vi "Set_Control_Parameter.vi"(0 "Set Mode":T18, 1 "Settings ok? in":bool, 5 "Settings message":T16, 7 "Main Parameters in":T1={"Mode"={"Mode"=enum."Dialog", "Expert?"=FALSE, "Dialog?"=FALSE}, "Stop loop"={"Settings changed?"=FALSE, "Stop?"=refnum}, "Send message"={"Send mode"=enum."Get parameters", "Set parameter list"=0, "Get parameter list"=0, "Reset device"=0, "Length set settings message"=0, "Reset buttons?"=FALSE, "Reset Master?"=enum."General"}, "Write settings"={"Options"=enum."File 1"}, "Settings state"={"MAS locked?"=refnum, "SLV locked?"=refnum}, "Button refs"={"Stop program"=refnum, "Save settings"=refnum, "DAQ mode"=refnum, "Reset settings"=refnum, "Apply settings"=refnum, "Reset MAS"=refnum, "Reset SLV"=refnum, "Local DBase?"=refnum, "Last value DBase"=FALSE, "Database"=refnum, "Calibration"=refnum, "Save settings 2"=refnum}, "Update screen"={"Detector number"=0, "Hardware"=enum."None"}, "Files"={"Path config file"=path "", "Path def. ini file"=path "", "Path ini file 1"=path "", "Path ini file 2"=path "", "Path RBF file"=path ""}, "DB connection"={"connection reference"=refnum, "Connected?"=refnum, "ODBC Name"=""}, "Status_id"=refnum, "Time difference"=refnum, "Satellites"=refnum, "Alignment parameters"=refnum, "Page Statistics 2"=refnum, "Database"=refnum, "Page Statistics"=refnum} {"Update screen"."Detector number" format="%#.0f"; "Send message"."Reset device" format="%x"; "Send message"."Get parameter list" format="%x"; "Send message"."Set parameter list" format="%x"}, 9 "Control Parameter in":T15 {"Aux Byte Value" format="%02x"; "Max Real Value" format="%#_6e"; "Min Real Value" format="%#_6e"; "dReal/dByte" format="%#_6e"; "Byte Value" format="%02x"; "Identifier" format="%02x"}, 11 "Status/Errors in":refnum<vi>, 12 "Control Parameters [] in":T15[](array[typedef]) {"Aux Byte Value" format="%02x"; "Max Real Value" format="%#_6e"; "Min Real Value" format="%#_6e"; "dReal/dByte" format="%#_6e"; "Byte Value" format="%02x"; "Identifier" format="%02x"}, 14 "Set value from device (f)":bool) -> (3 "Settings ok? out":bool, 4 "Value Changed?":bool, 8 "Run twice?":bool, 10 "Control Parameter out":T15 {"Aux Byte Value" format="%02x"; "Max Real Value" format="%#_6e"; "Min Real Value" format="%#_6e"; "dReal/dByte" format="%#_6e"; "Byte Value" format="%02x"; "Identifier" format="%02x"}, 15 "Status/Errors out":refnum<vi>)   [LabVIEW 2010]
uses:
  Controls/Control_Parameters.ctl
  Controls/Master.ctl
  Controls/Set_Mode.ctl
  Controls/Settings_Message.ctl
  Controls/Setting.ctl
  Controls/Main_Parameters.ctl
  Controls/Mode.ctl
  Controls/Stop_Loop.ctl
  Controls/Send_Message.ctl
  Controls/Send_Message_Mode.ctl
  Controls/Write_Settings.ctl
  Controls/Write_Settings_Options.ctl
  Controls/Settings_State.ctl
  Controls/Button_Refs.ctl
  Controls/Update_Screen.ctl
  Controls/Files.ctl
  Controls/DB_Connection.ctl
  database/Connection.llb/Conn ObjectReference.ctl
  Controls/TabPage_TriggerConditon.ctl
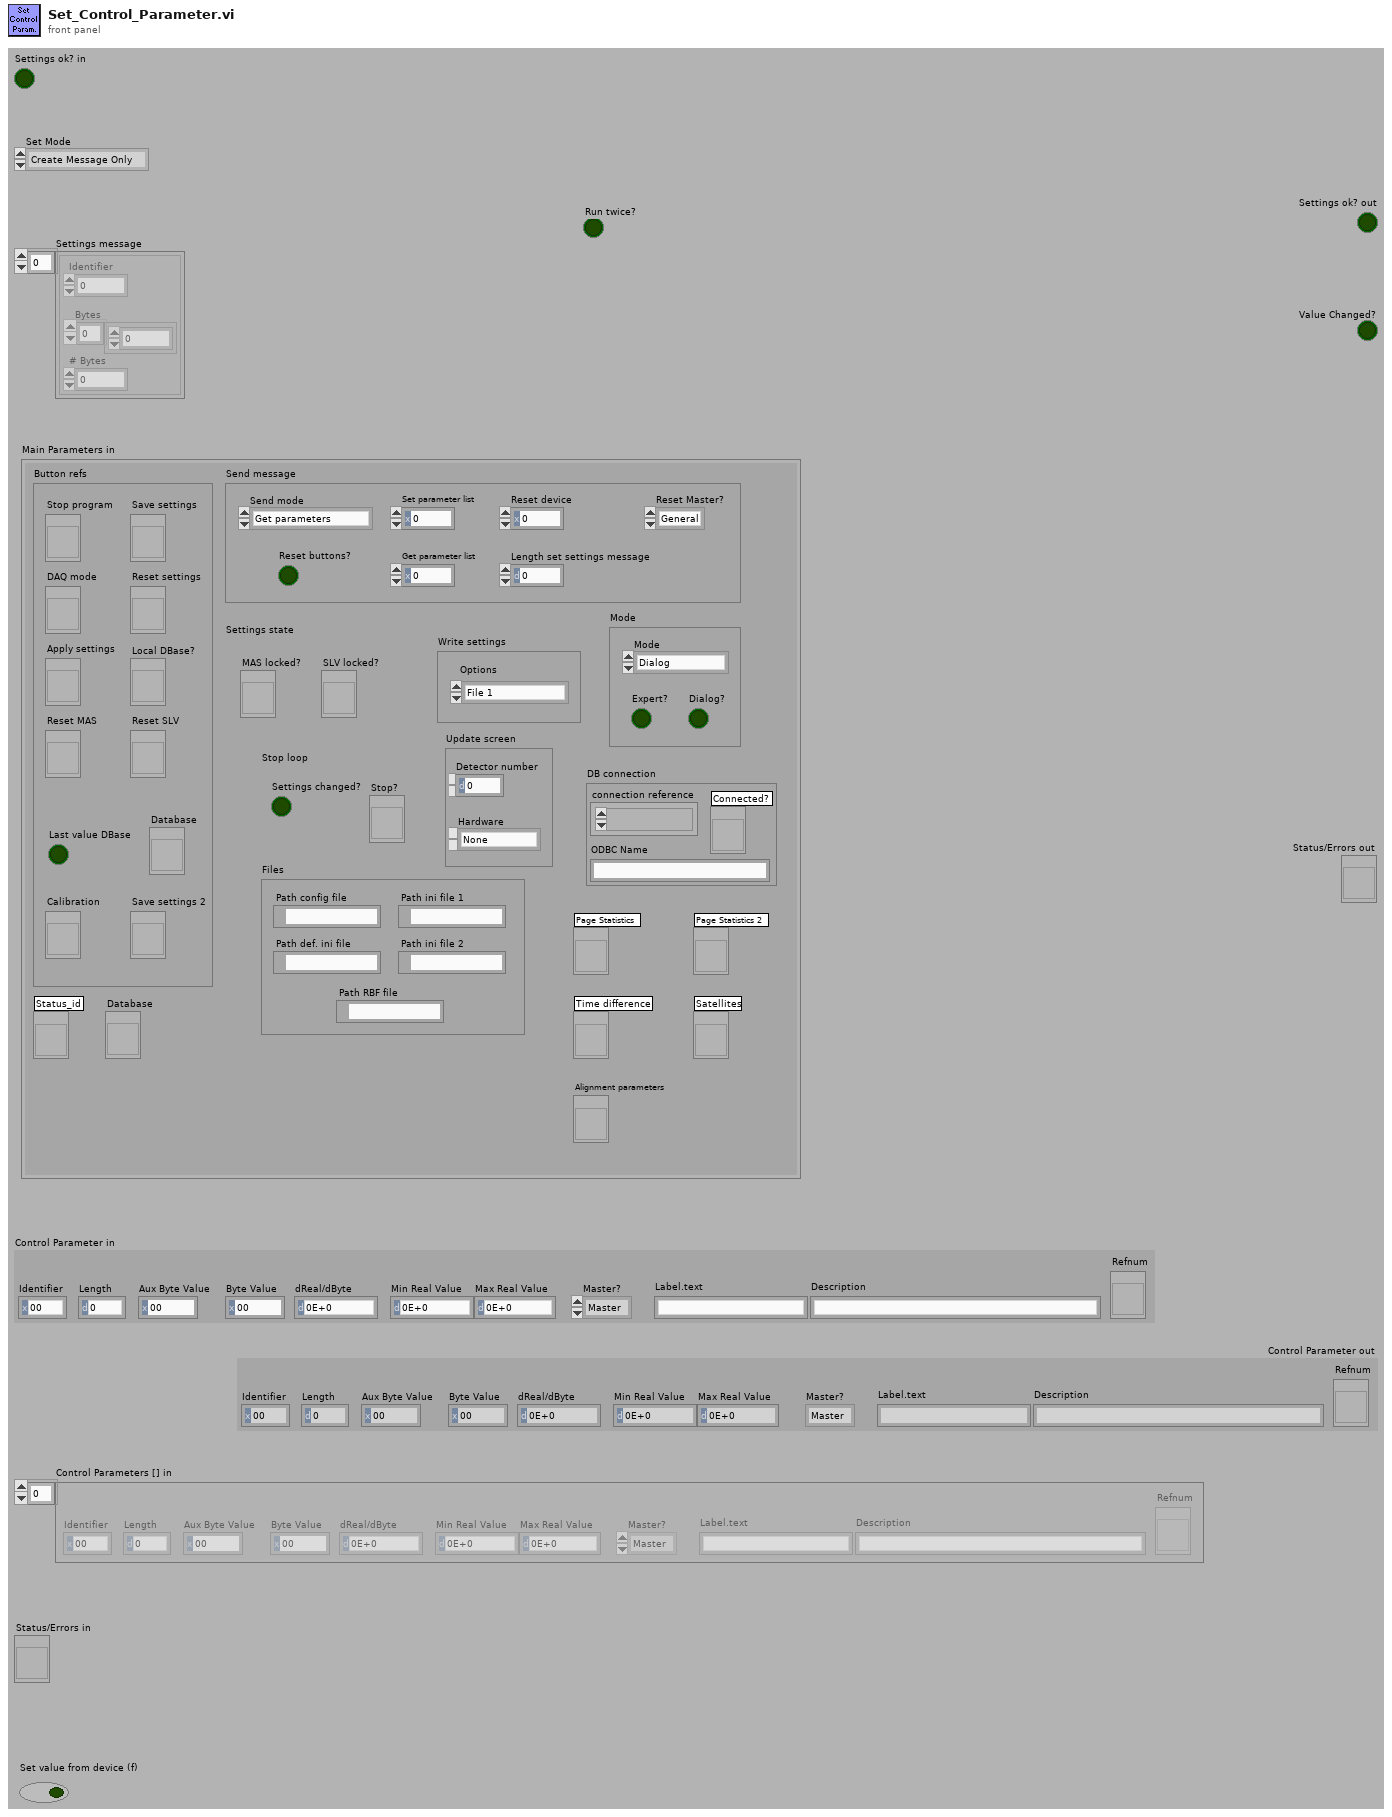
[diagram p1: front panel]
types:
  T1 = typedef "Main_Parameters.ctl" = cluster{"Mode":T2, "Stop loop":T3, "Send message":T4, "Write settings":T7, "Settings state":T9, "Button refs":T10, "Update screen":T11, "Files":T12, "DB connection":T13, "Status_id":refnum<vi>, "Time difference":refnum<vi>, "Satellites":refnum<vi>, "Alignment parameters":refnum<vi>, "Page Statistics 2":refnum<vi>, "Database":refnum<vi>, "Page Statistics":refnum<vi>}
  T2 = typedef "Mode.ctl" = cluster{"Mode":enum8{"Stop", "Dialog", "Hisparc II", "Hisparc II DAQ", "Alignment"}, "Expert?":bool, "Dialog?":bool}
  T3 = typedef "Stop_Loop.ctl" = cluster{"Settings changed?":bool, "Stop?":refnum<vi>}
  T4 = typedef "Send_Message.ctl" = cluster{"Send mode":T5, "Set parameter list":u8, "Get parameter list":u8, "Reset device":u8, "Length set settings message":i32, "Reset buttons?":bool, "Reset Master?":T6}
  T5 = typedef "Send_Message_Mode.ctl" = enum16{"Get parameters", "Set parameters", "From front panel", "From parameters", "Reset device", "Alignment"}
  T6 = typedef "Master.ctl" = enum16{"Master", "Slave", "General"}
  T7 = typedef "Write_Settings.ctl" = cluster{"Options":T8}
  T8 = typedef "Write_Settings_Options.ctl" = enum16{"File 1", "File 2", "Alignment", "Reset"}
  T9 = typedef "Settings_State.ctl" = cluster{"MAS locked?":refnum<vi>, "SLV locked?":refnum<vi>}
  T10 = typedef "Button_Refs.ctl" = cluster{"Stop program":refnum<vi>, "Save settings":refnum<vi>, "DAQ mode":refnum<vi>, "Reset settings":refnum<vi>, "Apply settings":refnum<vi>, "Reset MAS":refnum<vi>, "Reset SLV":refnum<vi>, "Local DBase?":refnum<vi>, "Last value DBase":bool, "Database":refnum<vi>, "Calibration":refnum<vi>, "Save settings 2":refnum<vi>}
  T11 = typedef "Update_Screen.ctl" = cluster{"Detector number":u16, "Hardware":enum8{"None", "HiSPARC I", "HiSPARC II", "HiSPARC III", "Unknown"}}
  T12 = typedef "Files.ctl" = cluster{"Path config file":path, "Path def. ini file":path, "Path ini file 1":path, "Path ini file 2":path, "Path RBF file":path}
  T13 = typedef "DB_Connection.ctl" = cluster{"connection reference":T14, "Connected?":refnum<vi>, "ODBC Name":string}
  T14 = typedef "Conn ObjectReference.ctl" = refnum<k1>
  T15 = typedef "Control_Parameters.ctl" = cluster{"Identifier":u8, "Length":u16, "Byte Value":u32, "dReal/dByte":dbl, "Min Real Value":dbl, "Max Real Value":dbl, "Master?":T6, "Label.text":string, "Description":string, "Refnum":refnum<vi>, "Aux Byte Value":u32}
  T16 = typedef "Settings_Message.ctl" = T17[]
  T17 = typedef "Setting.ctl" = cluster{"Identifier":u8, "  Bytes":u8[], "# Bytes":u16}
  T18 = typedef "Set_Mode.ctl" = enum16{"Create Message Only", "Front Panel", "Parameters", "Master", "Slave"}
  T19 = cluster{"Filter_Data":bool, "Use_Thresh":bool, "Reduce data?":bool}
  T20 = typedef "TabPage_TriggerConditon.ctl" = cluster{"# low signals":enum32{"no low", "1 low", "2 low", "3 low", "4 low"}, "# high signals":enum32{"no high", "1 high", "2 high", "3 high", "4 high"}, "External trigger":enum32{"no ext", "with ext", "only ext"}, "And_Or":cluster{"Switch":bool}}
  T21 = enum32{"no low", "1 low", "2 low", "3 low", "4 low"}
  T22 = enum32{"no high", "1 high", "2 high", "3 high", "4 high"}
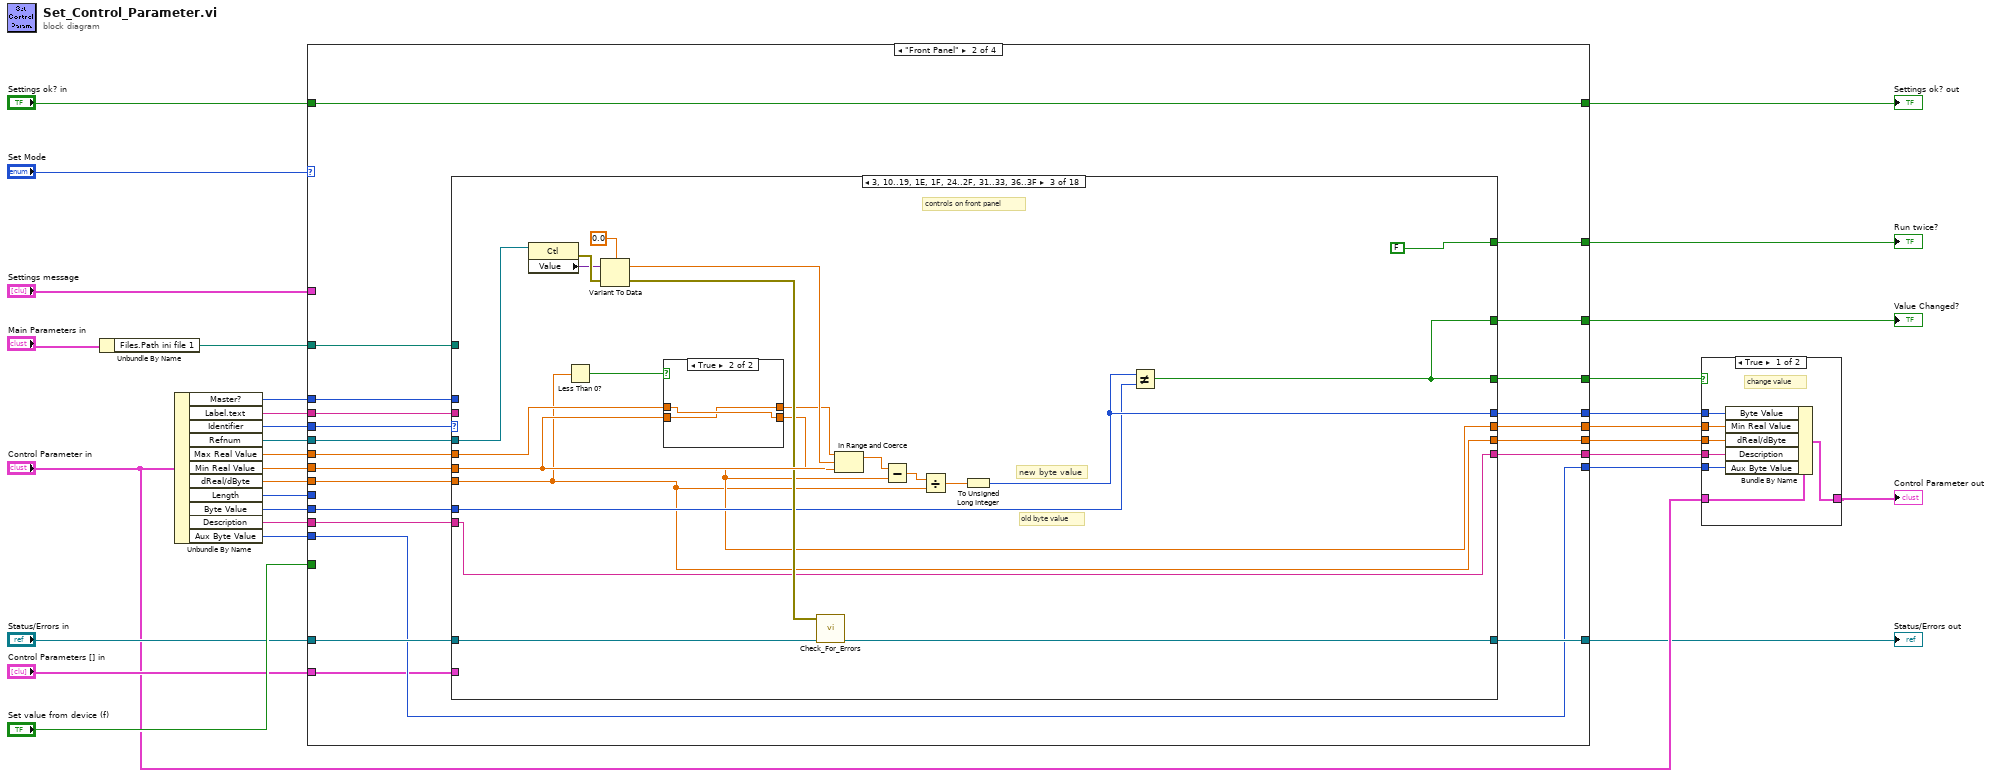
[diagram p0: block diagram]
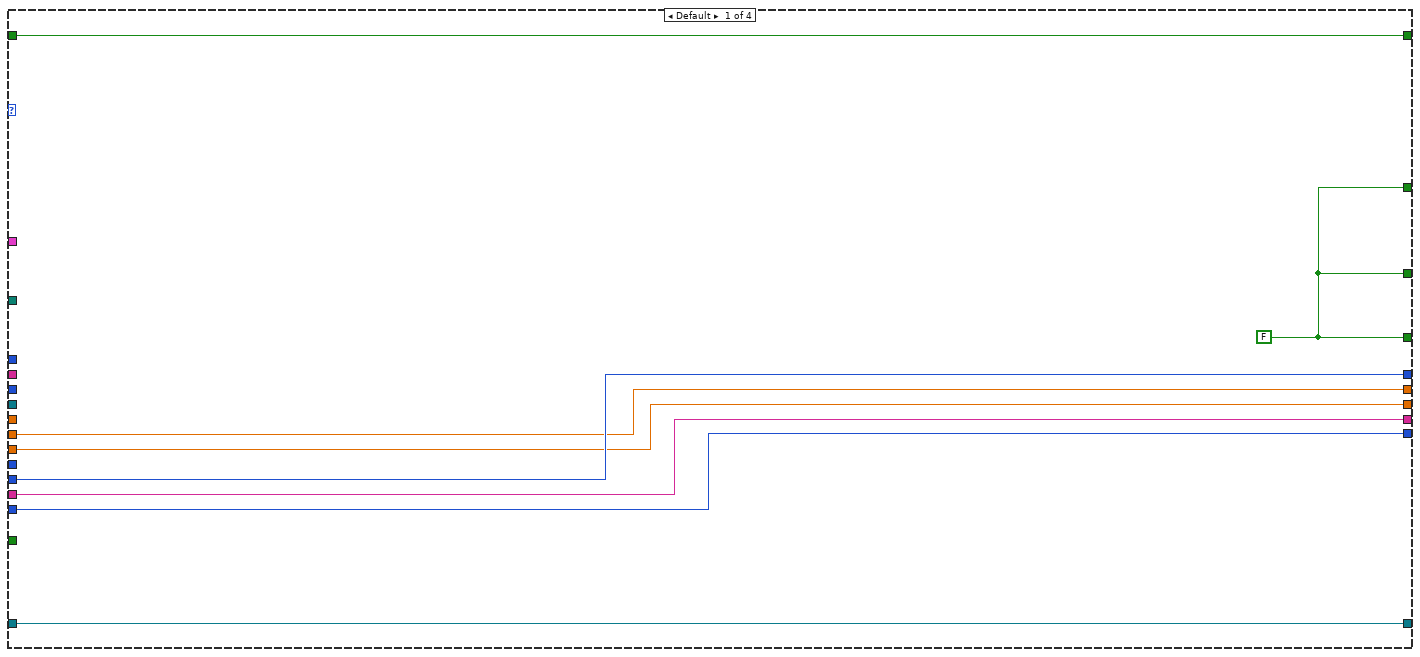
[diagram p3: hidden frame]
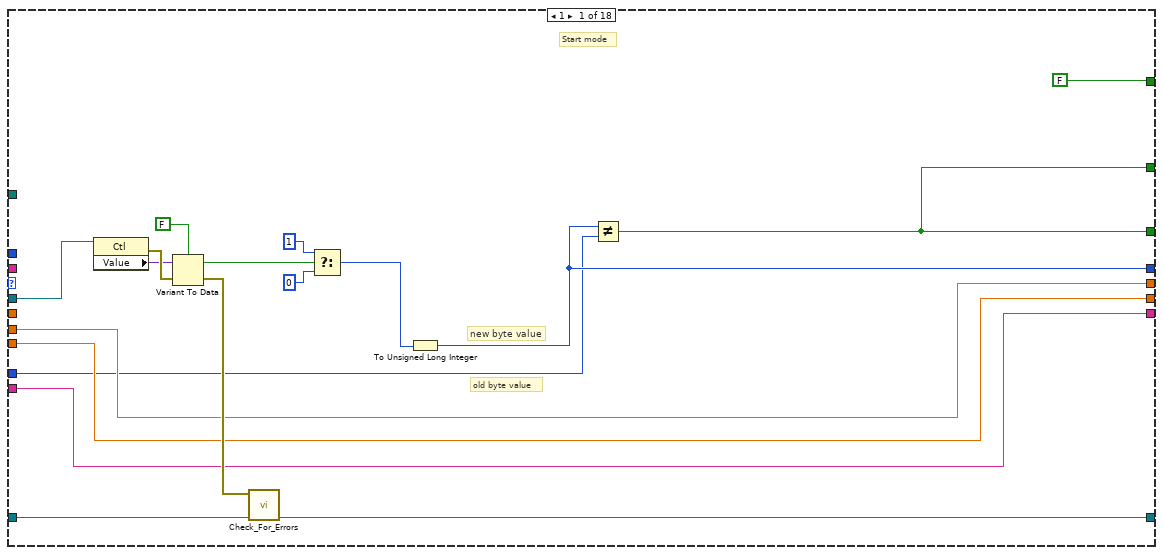
[diagram p4: hidden frame]
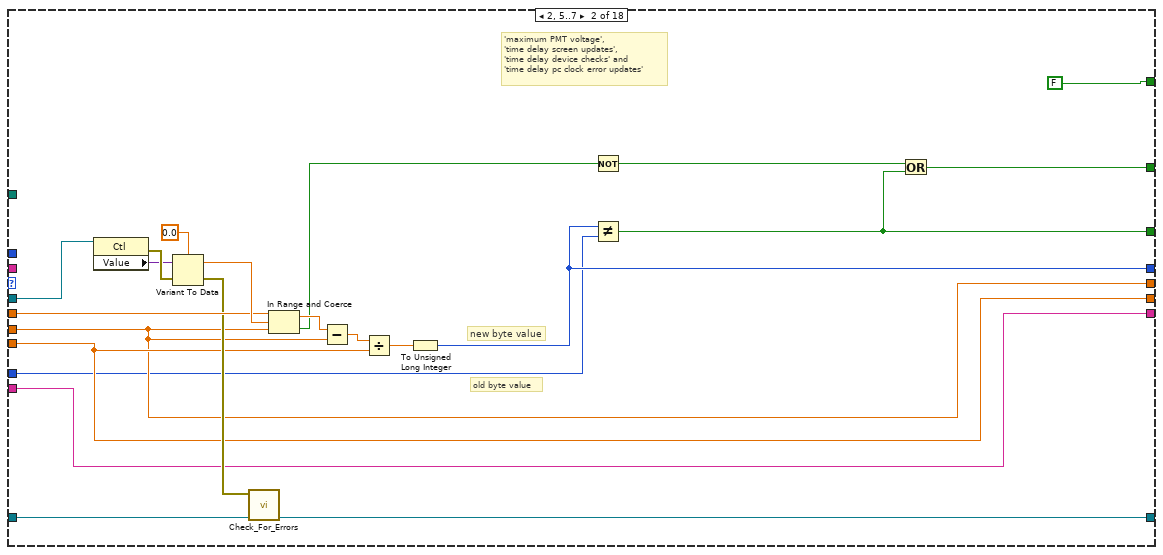
[diagram p5: hidden frame]
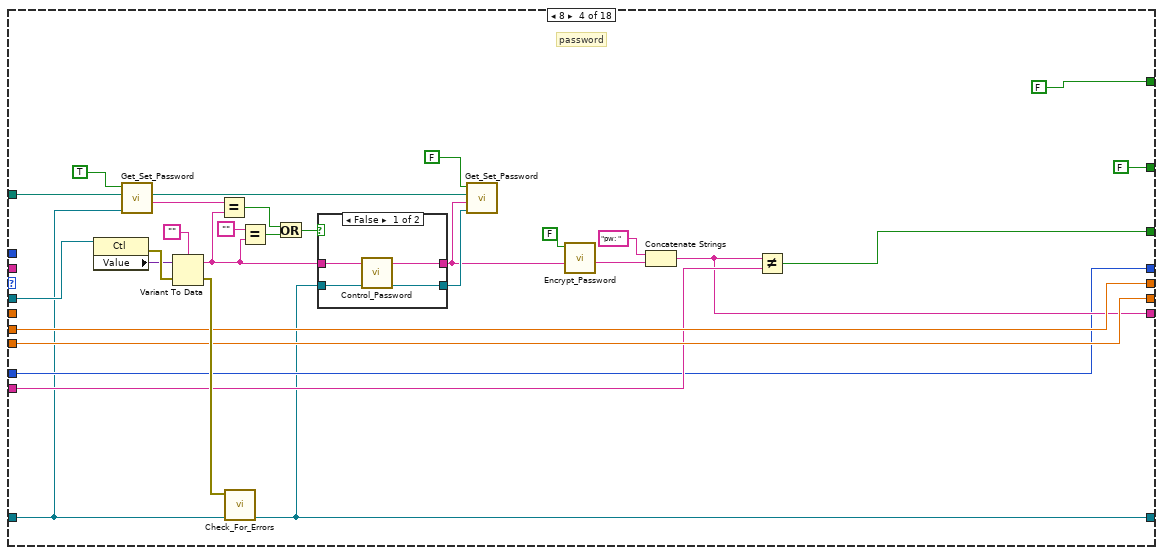
[diagram p7: hidden frame]
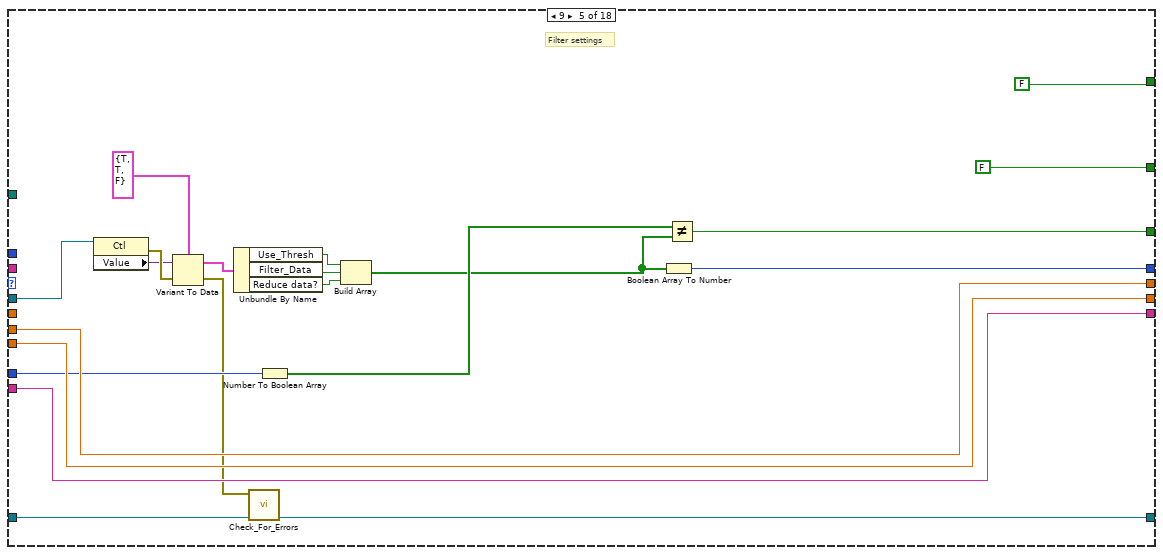
[diagram p9: hidden frame]
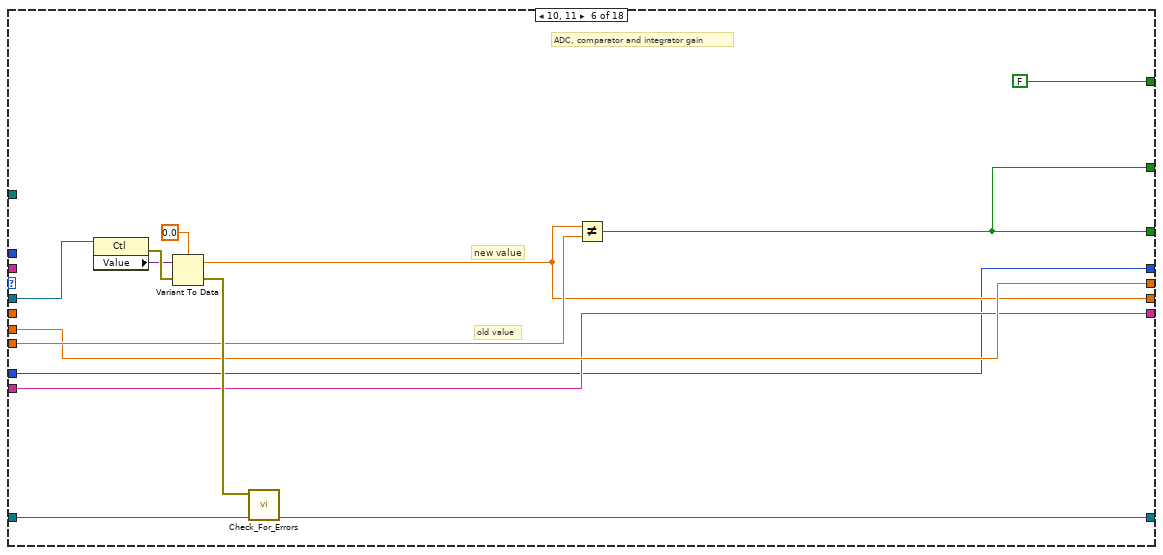
[diagram p10: hidden frame]
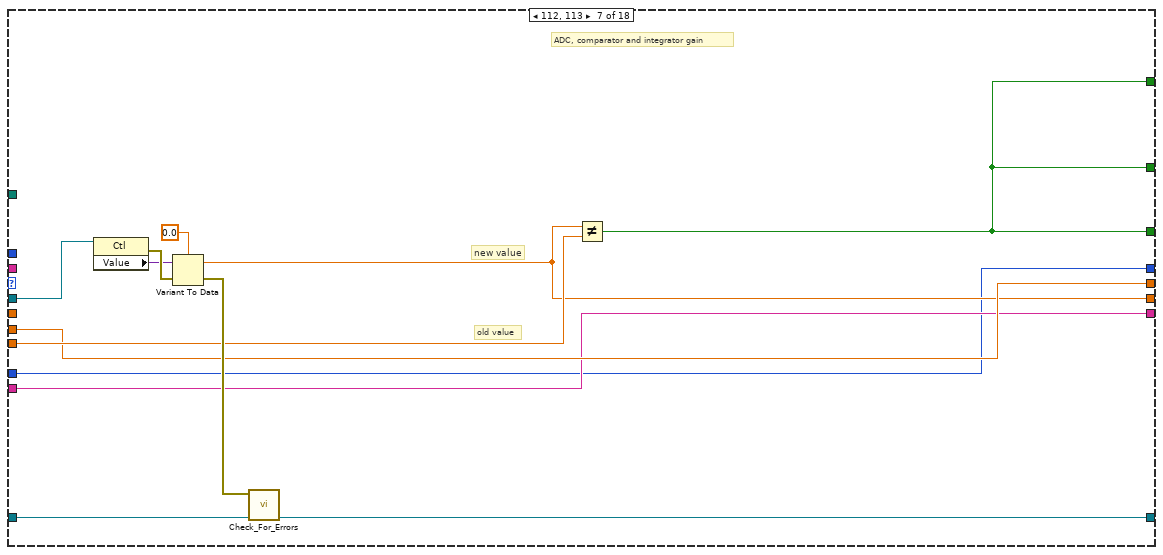
[diagram p11: hidden frame]
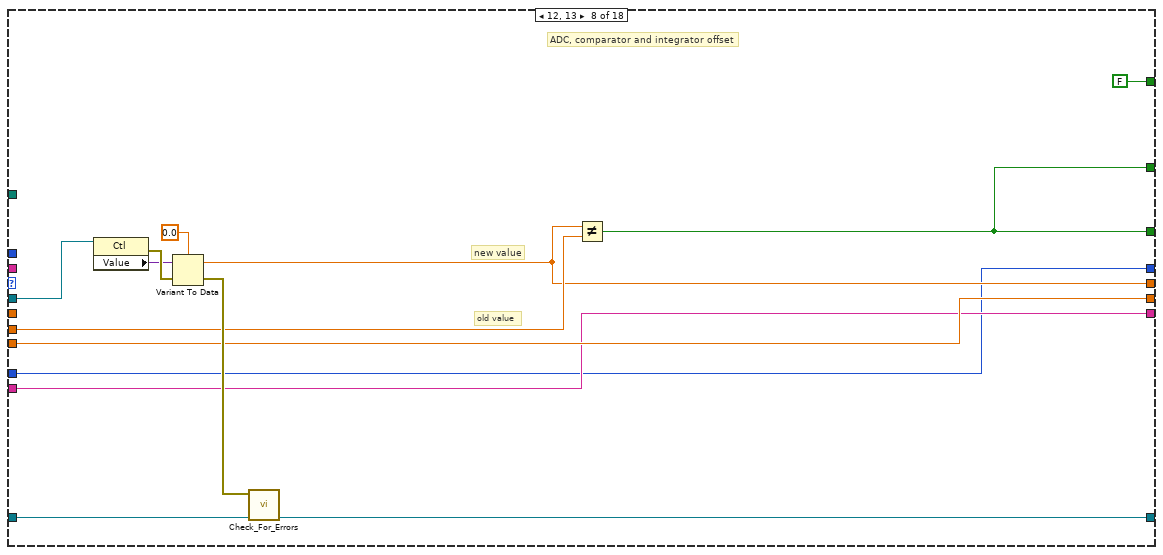
[diagram p12: hidden frame]
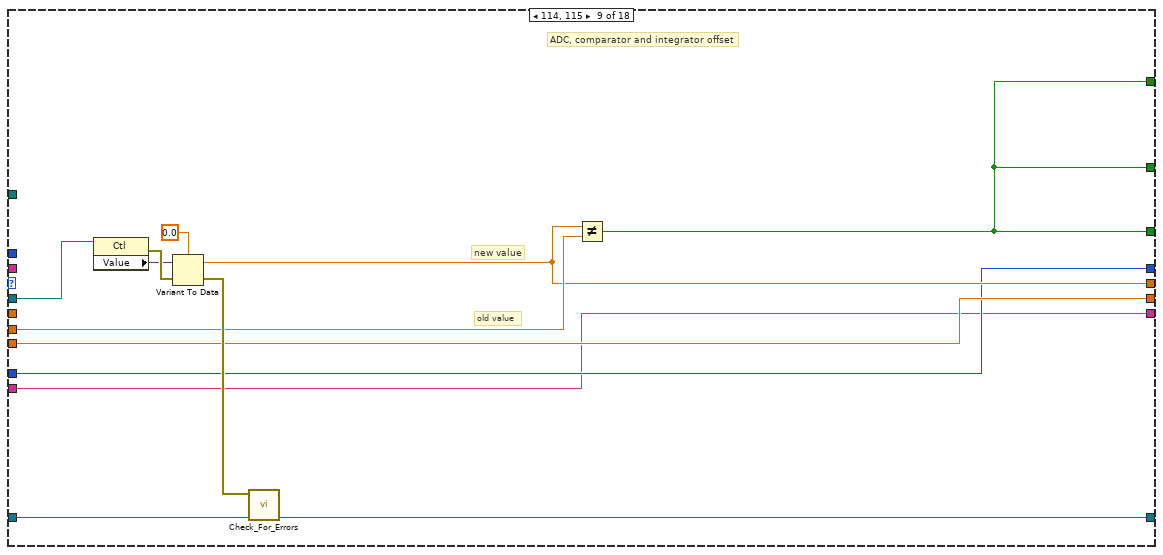
[diagram p13: hidden frame]
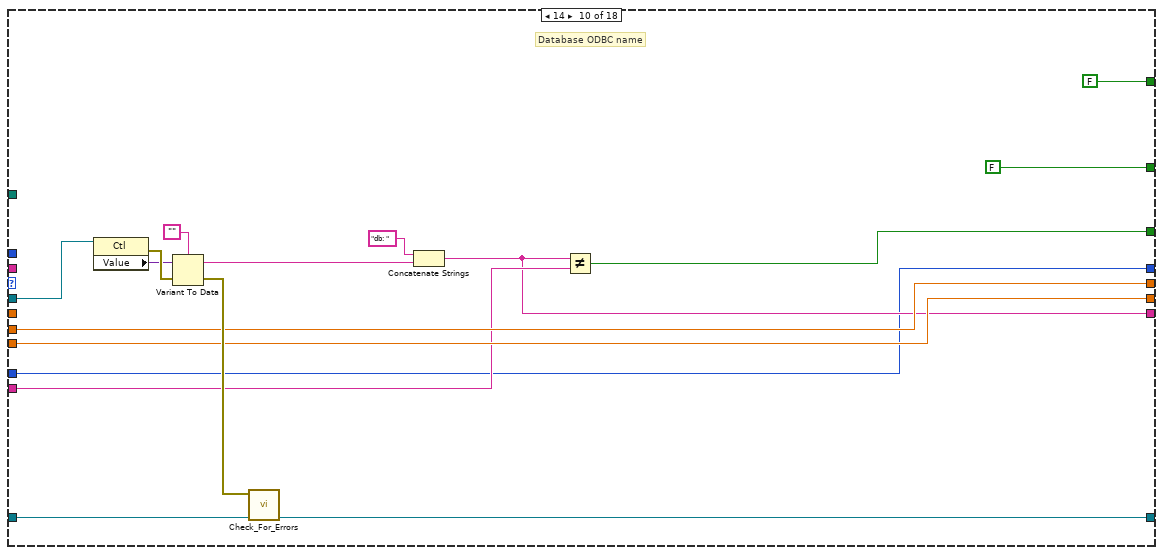
[diagram p14: hidden frame]
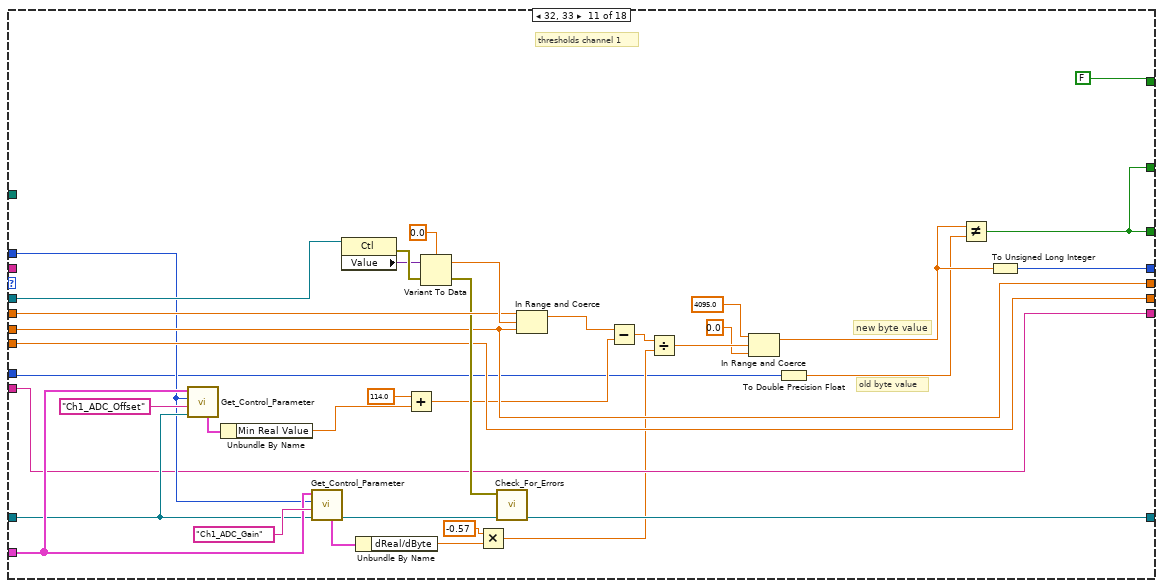
[diagram p15: hidden frame]
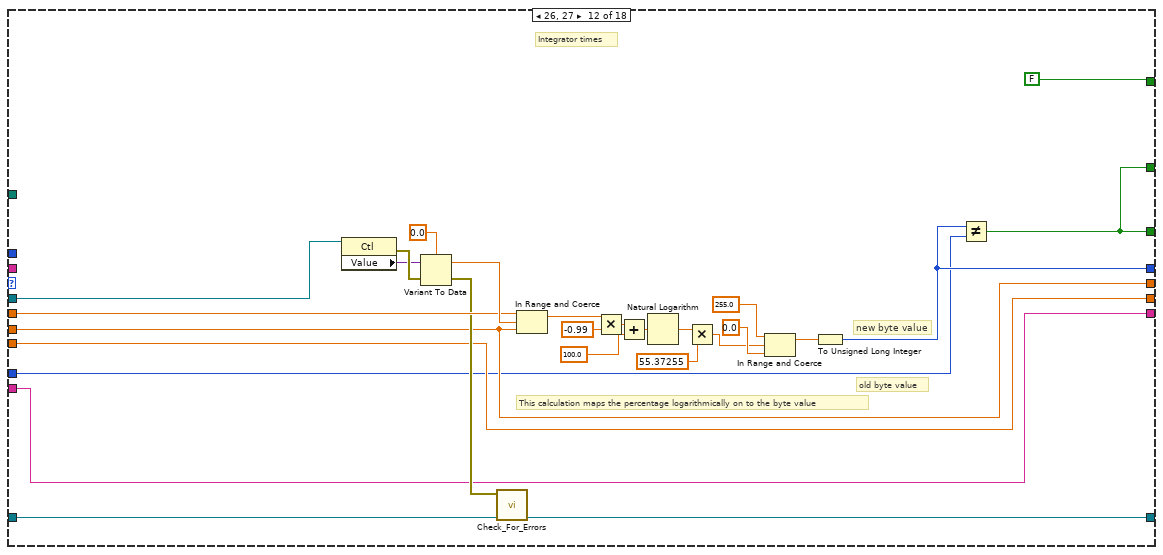
[diagram p16: hidden frame]
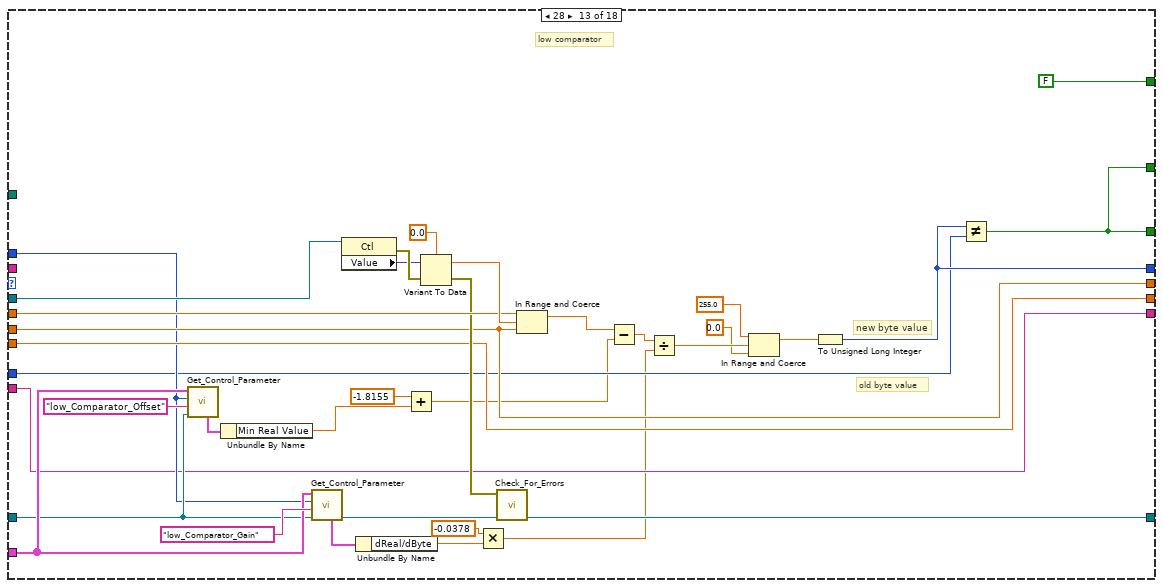
[diagram p17: hidden frame]
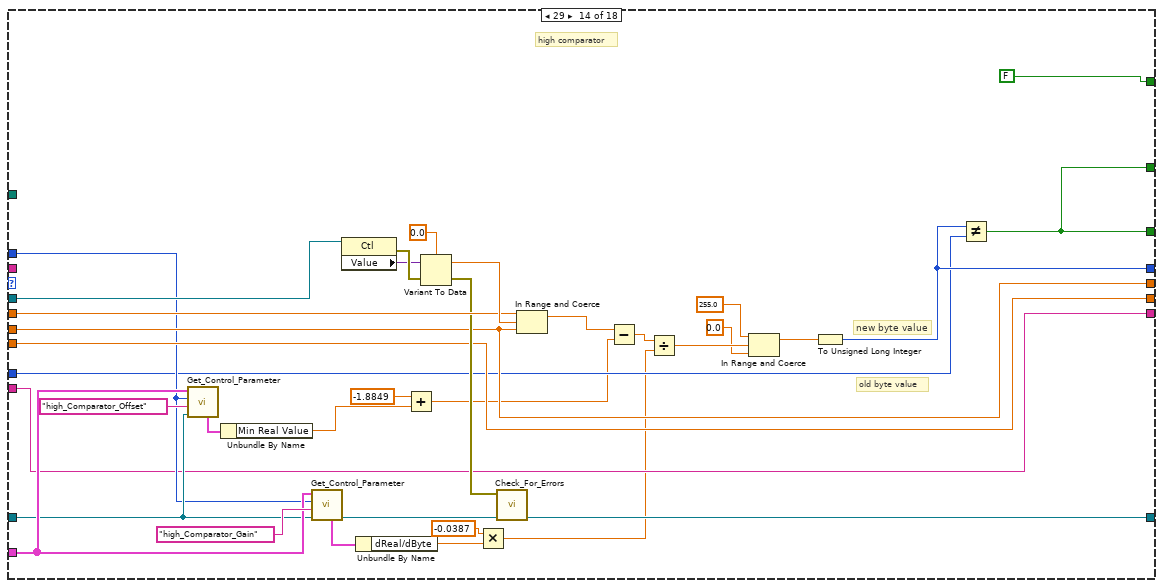
[diagram p18: hidden frame]
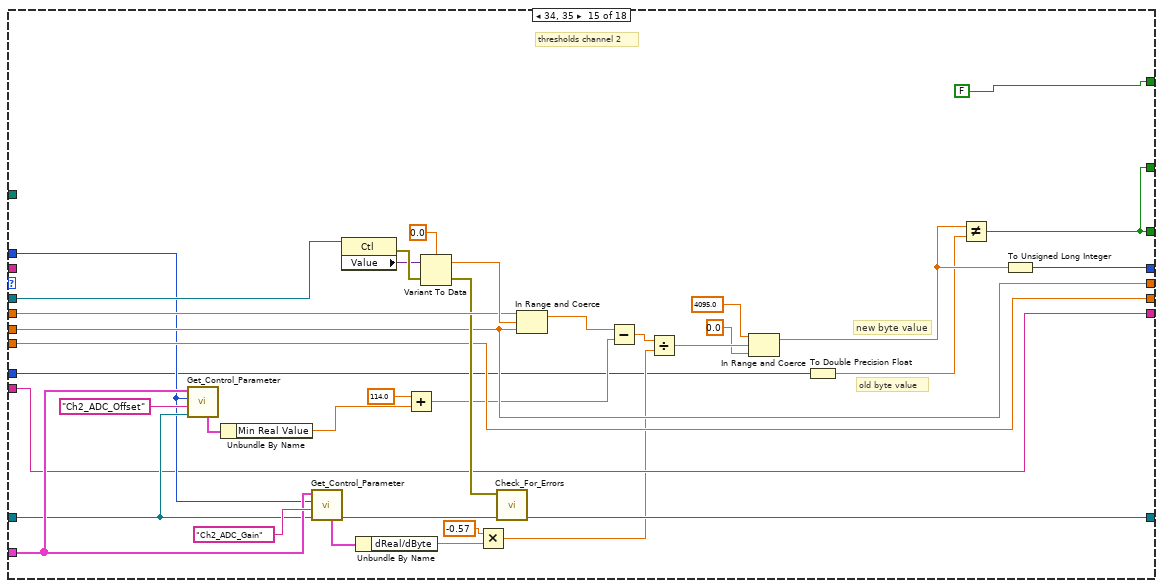
[diagram p19: hidden frame]
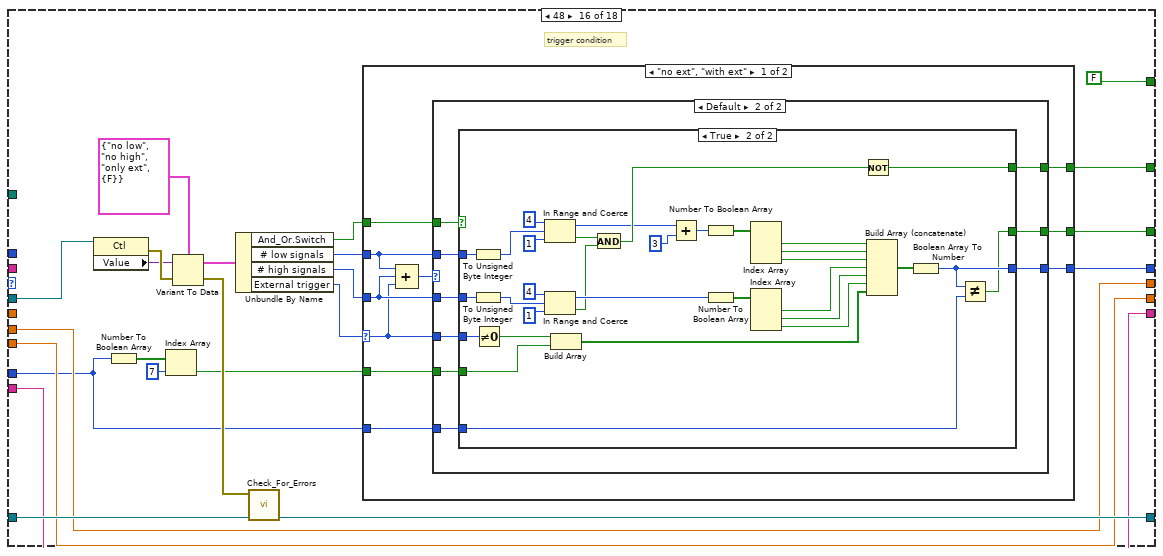
[diagram p20: hidden frame]
diagram:
  n1 = Unbundle By Name("Main Parameters in") -> ("Files.Path ini file 1"=w5:path)
  n2 = Unbundle By Name("Control Parameter in") -> ("Master?"=w24:T6, "Label.text"=w23:string, "Identifier"=w22:u8, "Refnum"=w21:refnum<vi>, "Max Real Value"=w20:dbl, "Min Real Value"=w19:dbl, "dReal/dByte"=w18:dbl, "Length"=w17:u16, "Byte Value"=w16:u32, "Description"=w15:string, "Aux Byte Value"=w14:u32)
  n3 = case shown="\"Front Panel\"" "Set Mode" {
    selector: "Set Mode" -> [_ _ w582 w855]
    tunnel: w19 -> [w34 w61 w567 w839]
    tunnel: w18 -> [w35 w60 w568 w840]
    tunnel: w16 -> [w39 w43 w585 w858]
    tunnel: [w38 w56 w578 w851] -> w1
    tunnel: w21 -> [_ w59 _ _]
    tunnel: w22 -> [_ w57 w574 w847]
    tunnel: w20 -> [_ w58 _ _]
    tunnel: "Settings message" -> [_ _ w584 w857]
    tunnel: w23 -> [_ w49 w581 w854]
    tunnel: w24 -> [_ w50 w580 w853]
    tunnel: [w39 w54 w579 w852] -> w30
    tunnel: [w32 w55 w570 w843] -> w28
    tunnel: "Status/Errors in" -> [w38 w53 w578 w851]
    tunnel: w17 -> [_ _ w577 w850]
    tunnel: [w37 w41 w576 w849] -> w3
    tunnel: "Settings ok? in" -> [w37 w41 w575 w848]
    tunnel: w14 -> [w36 w52 w572 w845]
    tunnel: [w36 w52 w571 w844] -> w29
    tunnel: [w32 w51 w570 w843] -> w4
    tunnel: "Set value from device (f)" -> [_ _ w569 w842]
    tunnel: [w34 w48 w567 w839] -> w27
    tunnel: [w35 w47 w568 w840] -> w25
    tunnel: "Control Parameters [] in" -> [_ w46 _ _]
    tunnel: w15 -> [w33 w45 w566 w841]
    tunnel: [w33 w44 w566 w841] -> w26
    tunnel: w5 -> [_ w42 _ _]
    tunnel: [w32 w40 FALSE FALSE] -> w2
    frame Default {
      w32 = FALSE
    }
    frame "Front Panel" {
      n4 = case shown="3, 10..19, 1E, 1F, 24..2F, 31..33, 36..3F" w57 {
        tunnel: w61 -> [w71 w83 w107 w151 w182 w190 w203 w218 w231 w247 w282 w309 w343 w378 w415 w429 w553 w563]
        tunnel: w60 -> [w70 w84 w105 w152 w183 w191 w204 w217 w230 w248 w281 w308 w342 w377 w414 w430 w554 w562]
        tunnel: w53 -> [w74 w91 w114 w140 w176 w193 w206 w220 w233 w250 w275 w302 w336 w371 w408 w443 w545 w564]
        tunnel: [w73 w85 w113 w141 w175 w192 w205 w219 w232 w249 w283 w311 w345 w380 w416 w442 w545 w564] -> w56
        tunnel: w59 -> [w76 w94 w116 w154 w174 w195 w208 w222 w235 w252 w286 w314 w348 w383 w419 w445 _ _]
        tunnel: w58 -> [_ w93 w106 _ _ _ _ _ _ _ w285 w313 w347 w382 w418 _ _ _]
        tunnel: [w65 w87 w102 w145 w167 w186 w199 w213 w226 w243 w260 w292 w319 w354 w393 w434 w558 w559] -> w55
        tunnel: [w72 w88 w112 w143 w168 w187 w200 w214 w228 w241 w259 w310 w344 w379 w392 w433 w556 w560] -> w54
        tunnel: [w65 w86 w102 FALSE FALSE w186 w199 w213 w226 FALSE w260 w292 w319 w354 w393 w435 FALSE w559] -> w51
        tunnel: w50 -> [_ _ _ _ _ _ _ _ _ _ w273 _ w334 w369 w406 _ _ _]
        tunnel: w49 -> [_ _ _ _ _ _ _ _ _ _ _ _ _ _ _ _ _ _]
        tunnel: [w71 w83 w107 w151 w182 w190 w203 w216 w229 w247 w282 w309 w343 w378 w415 w429 w553 w563] -> w48
        tunnel: [w70 w84 w105 w152 w183 w189 w202 w217 w230 w248 w281 w308 w342 w377 w414 w430 w554 w562] -> w47
        tunnel: w46 -> [_ _ _ _ _ _ _ _ _ _ w276 _ w337 w372 w409 _ _ _]
        tunnel: w45 -> [w64 w82 w111 w147 w181 w188 w201 w215 w227 w245 w272 w307 w333 w368 w405 w428 w548 w561]
        tunnel: [w64 w82 w111 w146 w181 w188 w201 w215 w227 w244 w272 w307 w333 w368 w405 w428 w548 w561] -> w44
        tunnel: w43 -> [w63 w81 w110 w143 w180 w187 w200 w214 w228 w241 w256 w306 w332 w367 w390 w427 w547 w560]
        tunnel: w42 -> [_ _ _ w138 _ _ _ _ _ _ _ _ _ _ _ _ _ _]
        tunnel: [FALSE FALSE FALSE FALSE FALSE FALSE w199 FALSE w226 FALSE FALSE FALSE FALSE FALSE FALSE FALSE FALSE w559] -> w40
        frame 1 {
          # "Start mode"
          # "old byte value"
          # "new byte value"
          n5 = property class="Ctl"(reference=w76) -> (error out=w79:errorcluster, "Value"=w78:variant)  [unwired: 1 in, 1 out]
          n6 = Variant To Data(error in=w79, Variant=w78, type=FALSE) -> (error out=w75:errorcluster, data=w69:bool)
          n7 = call "Check_For_Errors.vi"("Status/Errors in"=w74, "error in"=w75) -> ("Status/Errors out"=w73:refnum<vi>)  [unwired: 9 out]
          n8 = Select(t=u32 1 ("number"), s=w69, f=u32 0 ("number")) -> (s? t:f=w66:u32)
          n9 = To Unsigned Long Integer(number=w66) -> (unsigned 32bit integer=w72:u32)
          n10 = Not Equal?(x=w72, y=w63) -> (x != y?=w65:bool)
        }
        frame 2, 5..7 {
          # "old byte value"
          # "new byte value"
          # "'maximum PMT voltage',\n'time delay screen updates',\n'time delay device checks' and\n'time delay pc clock error updates'"
          n11 = property class="Ctl"(reference=w94) -> (error out=w101:errorcluster, "Value"=w100:variant)  [unwired: 1 in, 1 out]
          n12 = Variant To Data(error in=w101, Variant=w100, type=0.0 ("Byte Value")) -> (error out=w92:errorcluster, data=w98:dbl)
          n13 = call "Check_For_Errors.vi"("Status/Errors in"=w91, "error in"=w92) -> ("Status/Errors out"=w85:refnum<vi>)  [unwired: 9 out]
          n14 = In Range and Coerce(upper limit=w93, x=w98, lower limit=w83) -> (coerced(x)=w97:dbl, In Range?=w89:bool)
          n15 = Subtract(x=w97, y=w83) -> (x-y=w96:dbl)
          n16 = Divide(x=w96, y=w84) -> (x/y=w95:dbl)
          n17 = To Unsigned Long Integer(number=w95) -> (unsigned 32bit integer=w88:u32)
          n18 = Not(x=w89) -> (.not. x?=w90:bool)
          n19 = Not Equal?(x=w88, y=w81) -> (x != y?=w87:bool)
          n20 = Or(x=w90, y=w87) -> (x .or. y?=w86:bool)
        }
        frame 3, 16..25, 30, 31, 36..47, 49..51, 54..63 {
          # "old byte value"
          # "new byte value"
          # "controls on front panel"
          n21 = property class="Ctl"(reference=w116) -> (error out=w123:errorcluster, "Value"=w122:variant)  [unwired: 1 in, 1 out]
          n22 = Less Than 0?(x=w105) -> (x < 0?=w104:bool)
          n23 = Variant To Data(error in=w123, Variant=w122, type=0.0 ("Byte Value")) -> (error out=w115:errorcluster, data=w120:dbl)
          n24 = case shown="True" w104 {
            tunnel: w106 -> [w125 w127]
            tunnel: w107 -> [w124 w126]
            tunnel: [w124 w127] -> w108
            tunnel: [w125 w126] -> w109
            frame False {
            }
            frame True {
            }
          }
          n25 = call "Check_For_Errors.vi"("Status/Errors in"=w114, "error in"=w115) -> ("Status/Errors out"=w113:refnum<vi>)  [unwired: 9 out]
          n26 = In Range and Coerce(upper limit=w109, x=w120, lower limit=w108) -> (coerced(x)=w119:dbl)  [unwired: 1 out]
          n27 = Subtract(x=w119, y=w107) -> (x-y=w118:dbl)
          n28 = Divide(x=w118, y=w105) -> (x/y=w117:dbl)
          n29 = To Unsigned Long Integer(number=w117) -> (unsigned 32bit integer=w112:u32)
          n30 = Not Equal?(x=w112, y=w110) -> (x != y?=w102:bool)
        }
        frame 8 {
          # "password"
          n31 = property class="Ctl"(reference=w154) -> (error out=w157:errorcluster, "Value"=w156:variant)  [unwired: 1 in, 1 out]
          n32 = call "Get_Set_Password.vi"("Status/Errors in"=w140, "Path ini file in"=w138, "Get?"=TRUE) -> ("Password"=w139:string, "path"=w136:path)  [unwired: 1 in, 6 out]
          n33 = Variant To Data(error in=w157, Variant=w156, type="" ("Byte Value")) -> (error out=w153:errorcluster, data=w130:string)
          n34 = Equal?(x=w139, y=w130) -> (x = y?=w132:bool)
          n35 = call "Check_For_Errors.vi"("Status/Errors in"=w140, "error in"=w153) -> ("Status/Errors out"=w141:refnum<vi>)  [unwired: 9 out]
          n36 = Equal?(x="", y=w130) -> (x = y?=w129:bool)
          n37 = Or(x=w132, y=w129) -> (x .or. y?=w131:bool)
          n38 = case shown="False" w131 {
            tunnel: w130 -> [w159 w163]
            tunnel: [w158 w163] -> w133
            tunnel: w141 -> [w161 w162]
            tunnel: [w160 w162] -> w137
            frame False {
              n39 = call "Control_Password.vi"("Status/Errors in"=w161, "Password"=w159) -> ("Status/Errors out"=w160:refnum<vi>, "Password out"=w158:string)  [unwired: 2 in, 6 out]
            }
            frame True {
            }
          }
          n40 = call "Get_Set_Password.vi"("Status/Errors in"=w137, "Password"=w133, "Path ini file in"=w136, "Get?"=FALSE) -> ()  [unwired: 8 out]
          n41 = call "Encrypt_Password.vi"("Password in"=w133, "Decrypt?"=FALSE) -> ("Password out"=w149:string)  [unwired: 9 out]
          n42 = Concatenate Strings("pw: " ("string"), w149) -> (w146:string)
          n43 = Not Equal?(x=w146, y=w147) -> (x != y?=w145:bool)
        }
        frame 9 {
          # "Filter settings"
          n44 = property class="Ctl"(reference=w174) -> (error out=w179:errorcluster, "Value"=w178:variant)  [unwired: 1 in, 1 out]
          n45 = Variant To Data(error in=w179, Variant=w178, type=T19 {"Filter_Data"=TRUE, "Use_Thresh"=TRUE, "Reduce data?"=FALSE} ("Data_Filter")) -> (error out=w177:errorcluster, data=w172:T19)
          n46 = Unbundle By Name(w172) -> ("Use_Thresh"=w171:bool, "Filter_Data"=w170:bool, "Reduce data?"=w165:bool)
          n47 = call "Check_For_Errors.vi"("Status/Errors in"=w176, "error in"=w177) -> ("Status/Errors out"=w175:refnum<vi>)  [unwired: 9 out]
          n48 = Number To Boolean Array(number=w180) -> (Boolean array=w173:bool[])
          n49 = Build Array(w171, w170, w165) -> (w169:bool[])
          n50 = Boolean Array To Number(Boolean array=w169) -> (number=w168:u32)
          n51 = Not Equal?(x=w173, y=w169) -> (x != y?=w167:bool)
        }
        frame 10, 11 {
          # "old value"
          # "new value"
          # "ADC, comparator and integrator gain"
          n52 = property class="Ctl"(reference=w195) -> (error out=w198:errorcluster, "Value"=w197:variant)  [unwired: 1 in, 1 out]
          n53 = Variant To Data(error in=w198, Variant=w197, type=0.0 ("Byte Value")) -> (error out=w194:errorcluster, data=w189:dbl)
          n54 = call "Check_For_Errors.vi"("Status/Errors in"=w193, "error in"=w194) -> ("Status/Errors out"=w192:refnum<vi>)  [unwired: 9 out]
          n55 = Not Equal?(x=w189, y=w191) -> (x != y?=w186:bool)
        }
        frame 112, 113 {
          # "old value"
          # "new value"
          # "ADC, comparator and integrator gain"
          n56 = property class="Ctl"(reference=w208) -> (error out=w211:errorcluster, "Value"=w210:variant)  [unwired: 1 in, 1 out]
          n57 = Variant To Data(error in=w211, Variant=w210, type=0.0 ("Byte Value")) -> (error out=w207:errorcluster, data=w202:dbl)
          n58 = call "Check_For_Errors.vi"("Status/Errors in"=w206, "error in"=w207) -> ("Status/Errors out"=w205:refnum<vi>)  [unwired: 9 out]
          n59 = Not Equal?(x=w202, y=w204) -> (x != y?=w199:bool)
        }
        frame 12, 13 {
          # "old value"
          # "new value"
          # "ADC, comparator and integrator offset"
          n60 = property class="Ctl"(reference=w222) -> (error out=w225:errorcluster, "Value"=w224:variant)  [unwired: 1 in, 1 out]
          n61 = Variant To Data(error in=w225, Variant=w224, type=0.0 ("Byte Value")) -> (error out=w221:errorcluster, data=w216:dbl)
          n62 = call "Check_For_Errors.vi"("Status/Errors in"=w220, "error in"=w221) -> ("Status/Errors out"=w219:refnum<vi>)  [unwired: 9 out]
          n63 = Not Equal?(x=w216, y=w218) -> (x != y?=w213:bool)
        }
        frame 114, 115 {
          # "old value"
          # "new value"
          # "ADC, comparator and integrator offset"
          n64 = property class="Ctl"(reference=w235) -> (error out=w238:errorcluster, "Value"=w237:variant)  [unwired: 1 in, 1 out]
          n65 = Variant To Data(error in=w238, Variant=w237, type=0.0 ("Byte Value")) -> (error out=w234:errorcluster, data=w229:dbl)
          n66 = call "Check_For_Errors.vi"("Status/Errors in"=w233, "error in"=w234) -> ("Status/Errors out"=w232:refnum<vi>)  [unwired: 9 out]
          n67 = Not Equal?(x=w229, y=w231) -> (x != y?=w226:bool)
        }
        frame 14 {
          # "Database ODBC name"
          n68 = property class="Ctl"(reference=w252) -> (error out=w255:errorcluster, "Value"=w254:variant)  [unwired: 1 in, 1 out]
          n69 = Variant To Data(error in=w255, Variant=w254, type="" ("Byte Value")) -> (error out=w251:errorcluster, data=w240:string)
          n70 = call "Check_For_Errors.vi"("Status/Errors in"=w250, "error in"=w251) -> ("Status/Errors out"=w249:refnum<vi>)  [unwired: 9 out]
          n71 = Concatenate Strings("db: " ("string"), w240) -> (w244:string)
          n72 = Not Equal?(x=w244, y=w245) -> (x != y?=w243:bool)
        }
        frame 32, 33 {
          # "old byte value"
          # "new byte value"
          # "thresholds channel 1"
          n73 = call "Get_Control_Parameter.vi"("Status/Errors in"=w275, "Label.text in"="Ch1_ADC_Offset", "Master?"=w273, "Control Parameters [] in"=w276) -> ("Control Parameter"=w279:T15)  [unwired: 7 out]
          n74 = Unbundle By Name(w279) -> ("Min Real Value"=w265:dbl)
          n75 = call "Get_Control_Parameter.vi"("Status/Errors in"=w275, "Label.text in"="Ch1_ADC_Gain", "Master?"=w273, "Control Parameters [] in"=w276) -> ("Status/Errors out"=w274:refnum<vi>, "Control Parameter"=w277:T15)  [unwired: 6 out]
          n76 = property class="Ctl"(reference=w286) -> (error out=w291:errorcluster, "Value"=w290:variant)  [unwired: 1 in, 1 out]
          n77 = Unbundle By Name(w277) -> ("dReal/dByte"=w268:dbl)
          n78 = Add(x=114.0, y=w265) -> (x+y=w264:dbl)
          n79 = Variant To Data(error in=w291, Variant=w290, type=0.0 ("Byte Value")) -> (error out=w284:errorcluster, data=w288:dbl)
          n80 = Multiply(x=-0.57, y=w268) -> (x*y=w267:dbl)
          n81 = call "Check_For_Errors.vi"("Status/Errors in"=w274, "error in"=w284) -> ("Status/Errors out"=w283:refnum<vi>)  [unwired: 9 out]
          n82 = In Range and Coerce(upper limit=w285, x=w288, lower limit=w282) -> (coerced(x)=w262:dbl)  [unwired: 1 out]
          n83 = Subtract(x=w262, y=w264) -> (x-y=w287:dbl)
          n84 = Divide(x=w287, y=w267) -> (x/y=w271:dbl)
          n85 = In Range and Coerce(upper limit=4095.0, x=w271, lower limit=0.0 ("upper limit")) -> (coerced(x)=w258:dbl)  [unwired: 1 out]
          n86 = To Double Precision Float(number=w256) -> (double precision float=w257:dbl)
          n87 = Not Equal?(x=w258, y=w257) -> (x != y?=w260:bool)
          n88 = To Unsigned Long Integer(number=w258) -> (unsigned 32bit integer=w259:u32)
        }
        frame 26, 27 {
          # "This calculation maps the percentage logarithmically on to the byte value"
          # "old byte value"
          # "new byte value"
          # "Integrator times"
          n89 = property class="Ctl"(reference=w314) -> (error out=w318:errorcluster, "Value"=w317:variant)  [unwired: 1 in, 1 out]
          n90 = Variant To Data(error in=w318, Variant=w317, type=0.0 ("Byte Value")) -> (error out=w312:errorcluster, data=w315:dbl)
          n91 = call "Check_For_Errors.vi"("Status/Errors in"=w302, "error in"=w312) -> ("Status/Errors out"=w311:refnum<vi>)  [unwired: 9 out]
          n92 = In Range and Coerce(upper limit=w313, x=w315, lower limit=w309) -> (coerced(x)=w301:dbl)  [unwired: 1 out]
          n93 = Multiply(x=w301, y=-0.99) -> (x*y=w299:dbl)
          n94 = Add(x=w299, y=100.0) -> (x+y=w297:dbl)
          n95 = Natural Logarithm(1:w297) -> (0:w296:dbl)
          n96 = Multiply(x=w296, y=55.37255 ("x")) -> (x*y=w294:dbl)
          n97 = In Range and Coerce(upper limit=255.0, x=w294, lower limit=0.0 ("upper limit")) -> (coerced(x)=w305:dbl)  [unwired: 1 out]
          n98 = To Unsigned Long Integer(number=w305) -> (unsigned 32bit integer=w310:u32)
          n99 = Not Equal?(x=w310, y=w306) -> (x != y?=w292:bool)
        }
        frame 28 {
          # "old byte value"
          # "new byte value"
          # "low comparator"
          n100 = call "Get_Control_Parameter.vi"("Status/Errors in"=w336, "Label.text in"="low_Comparator_Offset", "Master?"=w334, "Control Parameters [] in"=w337) -> ("Control Parameter"=w340:T15)  [unwired: 7 out]
          n101 = Unbundle By Name(w340) -> ("Min Real Value"=w324:dbl)
          n102 = call "Get_Control_Parameter.vi"("Status/Errors in"=w336, "Label.text in"="low_Comparator_Gain", "Master?"=w334, "Control Parameters [] in"=w337) -> ("Status/Errors out"=w335:refnum<vi>, "Control Parameter"=w338:T15)  [unwired: 6 out]
          n103 = property class="Ctl"(reference=w348) -> (error out=w353:errorcluster, "Value"=w352:variant)  [unwired: 1 in, 1 out]
          n104 = Unbundle By Name(w338) -> ("dReal/dByte"=w327:dbl)
          n105 = Add(x=-1.8155, y=w324) -> (x+y=w323:dbl)
          n106 = Variant To Data(error in=w353, Variant=w352, type=0.0 ("Byte Value")) -> (error out=w346:errorcluster, data=w350:dbl)
          n107 = Multiply(x=-0.0378, y=w327) -> (x*y=w326:dbl)
          n108 = call "Check_For_Errors.vi"("Status/Errors in"=w335, "error in"=w346) -> ("Status/Errors out"=w345:refnum<vi>)  [unwired: 9 out]
          n109 = In Range and Coerce(upper limit=w347, x=w350, lower limit=w343) -> (coerced(x)=w321:dbl)  [unwired: 1 out]
          n110 = Subtract(x=w321, y=w323) -> (x-y=w349:dbl)
          n111 = Divide(x=w349, y=w326) -> (x/y=w330:dbl)
          n112 = In Range and Coerce(upper limit=255.0, x=w330, lower limit=0.0 ("upper limit")) -> (coerced(x)=w331:dbl)  [unwired: 1 out]
          n113 = To Unsigned Long Integer(number=w331) -> (unsigned 32bit integer=w344:u32)
          n114 = Not Equal?(x=w344, y=w332) -> (x != y?=w319:bool)
        }
        frame 29 {
          # "old byte value"
          # "new byte value"
          # "high comparator"
          n115 = call "Get_Control_Parameter.vi"("Status/Errors in"=w371, "Label.text in"="high_Comparator_Offset", "Master?"=w369, "Control Parameters [] in"=w372) -> ("Control Parameter"=w375:T15)  [unwired: 7 out]
          n116 = Unbundle By Name(w375) -> ("Min Real Value"=w359:dbl)
          n117 = call "Get_Control_Parameter.vi"("Status/Errors in"=w371, "Label.text in"="high_Comparator_Gain", "Master?"=w369, "Control Parameters [] in"=w372) -> ("Status/Errors out"=w370:refnum<vi>, "Control Parameter"=w373:T15)  [unwired: 6 out]
          n118 = property class="Ctl"(reference=w383) -> (error out=w388:errorcluster, "Value"=w387:variant)  [unwired: 1 in, 1 out]
          n119 = Unbundle By Name(w373) -> ("dReal/dByte"=w362:dbl)
          n120 = Add(x=-1.8849, y=w359) -> (x+y=w358:dbl)
          n121 = Variant To Data(error in=w388, Variant=w387, type=0.0 ("Byte Value")) -> (error out=w381:errorcluster, data=w385:dbl)
          n122 = Multiply(x=-0.0387, y=w362) -> (x*y=w361:dbl)
          n123 = call "Check_For_Errors.vi"("Status/Errors in"=w370, "error in"=w381) -> ("Status/Errors out"=w380:refnum<vi>)  [unwired: 9 out]
          n124 = In Range and Coerce(upper limit=w382, x=w385, lower limit=w378) -> (coerced(x)=w356:dbl)  [unwired: 1 out]
          n125 = Subtract(x=w356, y=w358) -> (x-y=w384:dbl)
          n126 = Divide(x=w384, y=w361) -> (x/y=w365:dbl)
          n127 = In Range and Coerce(upper limit=255.0, x=w365, lower limit=0.0 ("upper limit")) -> (coerced(x)=w366:dbl)  [unwired: 1 out]
          n128 = To Unsigned Long Integer(number=w366) -> (unsigned 32bit integer=w379:u32)
          n129 = Not Equal?(x=w379, y=w367) -> (x != y?=w354:bool)
        }
        frame 34, 35 {
          # "old byte value"
          # "new byte value"
          # "thresholds channel 2"
          n130 = call "Get_Control_Parameter.vi"("Status/Errors in"=w408, "Label.text in"="Ch2_ADC_Offset", "Master?"=w406, "Control Parameters [] in"=w409) -> ("Control Parameter"=w412:T15)  [unwired: 7 out]
          n131 = Unbundle By Name(w412) -> ("Min Real Value"=w398:dbl)
          n132 = call "Get_Control_Parameter.vi"("Status/Errors in"=w408, "Label.text in"="Ch2_ADC_Gain", "Master?"=w406, "Control Parameters [] in"=w409) -> ("Status/Errors out"=w407:refnum<vi>, "Control Parameter"=w410:T15)  [unwired: 6 out]
          n133 = property class="Ctl"(reference=w419) -> (error out=w424:errorcluster, "Value"=w423:variant)  [unwired: 1 in, 1 out]
          n134 = Unbundle By Name(w410) -> ("dReal/dByte"=w401:dbl)
          n135 = Add(x=114.0, y=w398) -> (x+y=w397:dbl)
          n136 = Variant To Data(error in=w424, Variant=w423, type=0.0 ("Byte Value")) -> (error out=w417:errorcluster, data=w421:dbl)
          n137 = Multiply(x=-0.57, y=w401) -> (x*y=w400:dbl)
          n138 = call "Check_For_Errors.vi"("Status/Errors in"=w407, "error in"=w417) -> ("Status/Errors out"=w416:refnum<vi>)  [unwired: 9 out]
          n139 = In Range and Coerce(upper limit=w418, x=w421, lower limit=w415) -> (coerced(x)=w395:dbl)  [unwired: 1 out]
          n140 = Subtract(x=w395, y=w397) -> (x-y=w420:dbl)
          n141 = Divide(x=w420, y=w400) -> (x/y=w404:dbl)
          n142 = In Range and Coerce(upper limit=4095.0, x=w404, lower limit=0.0 ("upper limit")) -> (coerced(x)=w391:dbl)  [unwired: 1 out]
          n143 = To Double Precision Float(number=w390) -> (double precision float=w389:dbl)
          n144 = Not Equal?(x=w391, y=w389) -> (x != y?=w393:bool)
          n145 = To Unsigned Long Integer(number=w391) -> (unsigned 32bit integer=w392:u32)
        }
        frame 48 {
          # "trigger condition"
          n146 = property class="Ctl"(reference=w445) -> (error out=w447:errorcluster, "Value"=w446:variant)  [unwired: 1 in, 1 out]
          n147 = Number To Boolean Array(number=w427) -> (Boolean array=w439:bool[])
          n148 = Index Array(array=w439, index=7) -> (element=w432:bool)
          n149 = Variant To Data(error in=w447, Variant=w446, type=T20 {"# low signals"=enum."no low", "# high signals"=enum."no high", "External trigger"=enum."only ext", "And_Or"={"Switch"=FALSE}} ("Trigger Condition")) -> (error out=w444:errorcluster, data=w440:T20)
          n150 = Unbundle By Name(w440) -> ("And_Or.Switch"=w426:bool, "# low signals"=w437:T21, "# high signals"=w436:T22, "External trigger"=w431:enum32{"no ext", "with ext", "only ext"})
          n151 = call "Check_For_Errors.vi"("Status/Errors in"=w443, "error in"=w444) -> ("Status/Errors out"=w442:refnum<vi>)  [unwired: 9 out]
          n152 = case shown="\"no ext\", \"with ext\"" w431 {
            selector: w431 -> [w448 _]
            tunnel: w436 -> [w450 w533]
            tunnel: w437 -> [w451 w532]
            tunnel: [w453 w540] -> w435
            tunnel: [w456 w535] -> w433
            tunnel: w427 -> [w457 w536]
            tunnel: [w455 w534] -> w434
            tunnel: w432 -> [w454 w539]
            tunnel: w426 -> [w452 _]
            frame "no ext", "with ext" {
              n153 = Compound Arithmetic op=unknown(w451, w450, w448) -> (w449:u32)
              n154 = case shown="Default" w449 {
                tunnel: w457 -> [w460 w473]
                tunnel: [w459 w472] -> w456
                tunnel: [w458 w471] -> w455
                tunnel: w450 -> [_ w470]
                tunnel: w451 -> [_ w469]
                tunnel: w454 -> [w461 w468]
                tunnel: w448 -> [_ w467]
                tunnel: [TRUE w466] -> w453
                tunnel: w452 -> [_ w465]
                frame 0 {
                  n155 = Select(t=u32 192, s=w461, f=u32 64) -> (s? t:f=w459:u32)
                  n156 = Not Equal?(x=w459, y=w460) -> (x != y?=w458:bool)
                }
                frame Default {
                  n157 = case shown="True" w465 {
                    tunnel: w473 -> [w491 w527]
                    tunnel: [w490 w526] -> w472
                    tunnel: [w489 w525] -> w471
                    tunnel: w470 -> [w487 w523]
                    tunnel: w469 -> [w485 w522]
                    tunnel: w468 -> [w483 w520]
                    tunnel: w467 -> [w475 w512]
                    tunnel: [w474 w511] -> w466
                    frame False {
                      n158 = To Unsigned Byte Integer(number=w485) -> (unsigned 8bit integer=w484:u8)
                      n159 = To Unsigned Byte Integer(number=w487) -> (unsigned 8bit integer=w486:u8)
                      n160 = Not Equal To 0?(x=w475) -> (x != 0?=w488:bool)
                      n161 = Build Array(w488, w483) -> (w482:bool[])
                      n162 = Subtract(x=u8 4, y=w486) -> (x-y=w498:u8)
                      n163 = In Range and Coerce(upper limit=w498, x=w484, lower limit=u8 0) -> (coerced(x)=w496:u8, In Range?=w495:bool)
                      n164 = Number To Boolean Array(number=w496) -> (Boolean array=w493:bool[])
                      n165 = Number To Boolean Array(number=w486) -> (Boolean array=w494:bool[])
                      n166 = Index Array(array=w493) -> (element #1=w476:bool, element #2=w477:bool, element #3=w478:bool)  [unwired: 3 in]
                      n167 = Index Array(array=w494) -> (element #1=w479:bool, element #2=w480:bool, element #3=w481:bool)  [unwired: 3 in]
                      n168 = Not(x=w495) -> (.not. x?=w474:bool)
                      n169 = Build Array (concatenate)(w476, w477, w478, w479, w480, w481, w482) -> (w492:bool[])
                      n170 = Boolean Array To Number(Boolean array=w492) -> (number=w490:u32)
                      n171 = Not Equal?(x=w490, y=w491) -> (x != y?=w489:bool)
                    }
                    frame True {
                      n172 = To Unsigned Byte Integer(number=w522) -> (unsigned 8bit integer=w521:u8)
                      n173 = To Unsigned Byte Integer(number=w523) -> (unsigned 8bit integer=w506:u8)
                      n174 = Not Equal To 0?(x=w512) -> (x != 0?=w524:bool)
                      n175 = In Range and Coerce(upper limit=u8 4, x=w521, lower limit=u8 1) -> (coerced(x)=w501:u8, In Range?=w505:bool)
                      n176 = In Range and Coerce(upper limit=u8 4, x=w506, lower limit=u8 1) -> (coerced(x)=w507:u8, In Range?=w504:bool)
                      n177 = Build Array(w524, w520) -> (w519:bool[])
                      n178 = And(x=w505, y=w504) -> (x .and. y?=w503:bool)
                      n179 = Add(x=w501, y=u8 3) -> (x+y=w502:u8)
                      n180 = Number To Boolean Array(number=w502) -> (Boolean array=w529:bool[])
                      n181 = Number To Boolean Array(number=w507) -> (Boolean array=w530:bool[])
                      n182 = Index Array(array=w529) -> (element #1=w513:bool, element #2=w514:bool, element #3=w515:bool)  [unwired: 3 in]
                      n183 = Index Array(array=w530) -> (element #1=w516:bool, element #2=w517:bool, element #3=w518:bool)  [unwired: 3 in]
                      n184 = Not(x=w503) -> (.not. x?=w511:bool)
                      n185 = Build Array (concatenate)(w513, w514, w515, w516, w517, w518, w519) -> (w528:bool[])
                      n186 = Boolean Array To Number(Boolean array=w528) -> (number=w526:u32)
                      n187 = Not Equal?(x=w526, y=w527) -> (x != y?=w525:bool)
                    }
                  }
                }
              }
            }
            frame "only ext" {
              n188 = Equal To 0?(x=w532) -> (x = 0?=w543:bool)
              n189 = Equal To 0?(x=w533) -> (x = 0?=w542:bool)
              n190 = And(x=w543, y=w542) -> (x .and. y?=w541:bool)
              n191 = Select(t=u32 192, s=w539, f=u32 64) -> (s? t:f=w535:u32)
              n192 = Not Equal?(x=w535, y=w536) -> (x != y?=w534:bool)
              n193 = Not(x=w541) -> (.not. x?=w540:bool)
            }
          }
        }
        frame 53 {
          # "Spare bytes:\nbit 0:  listing/writing mode\nbit 1:  second messages\nbit 2:  program GPS receiver\nbit 3:  master/slave state"
          n194 = Number To Boolean Array(number=w547) -> (Boolean array=w550:bool[])
          n195 = Replace Array Subset(array=w550, new element #1=TRUE ("new element/subarray"), new element #2=TRUE ("new element/subarray"), new element #3=TRUE ("new element/subarray"), new element #4=FALSE ("new element/subarray")) -> (w549:bool[])  [unwired: 4 in]
          n196 = Boolean Array To Number(Boolean array=w549) -> (number=w556:u32)
          n197 = Not Equal?(x=w550, y=w549) -> (x != y?=w558:bool)
        }
        frame 4, 52, Default {
          w559 = FALSE
          # "storage condition is updated in 'Handle_Buttons.vi'"
          # "storage condition (local DBase?), Status electronics, default"
          # "Status electronics is not connected\nto a control of which we can change the value."
        }
      }
    }
    frame "Master" {
      n198 = case shown="\"Master\"" w582 {
        tunnel: [FALSE w590 w599] -> w583
        tunnel: w581 -> [_ w589 w598]
        tunnel: w580 -> [_ w588 w597]
        frame Default {
        }
        frame "Master" {
          n199 = String Subset(string=w589, length (rest)=3 ("length (rest)")) -> (substring=w593:string)  [unwired: 1 out]
          n200 = Not Equal?(x=Master."Slave", y=w588) -> (x != y?=w594:bool)
          n201 = Not Equal?(x=w593, y="SLV") -> (x != y?=w595:bool)
          n202 = And(x=w594, y=w595) -> (x .and. y?=w590:bool)
        }
        frame "Slave" {
          n203 = String Subset(string=w598, length (rest)=3 ("length (rest)")) -> (substring=w602:string)  [unwired: 1 out]
          n204 = Not Equal?(x=Master."Master", y=w597) -> (x != y?=w603:bool)
          n205 = Not Equal?(x=w602, y="MAS") -> (x != y?=w604:bool)
          n206 = And(x=w603, y=w604) -> (x .and. y?=w599:bool)
        }
      }
      n207 = case shown="True" w583 {
        tunnel: w585 -> [w614 w836]
        tunnel: w574 -> [w613 _]
        tunnel: [w610 FALSE] -> w570
        tunnel: w584 -> [w612 _]
        tunnel: [w611 w836] -> w579
        tunnel: w577 -> [w609 _]
        tunnel: [w608 TRUE] -> w573
        tunnel: w572 -> [w607 w834]
        tunnel: [w606 w834] -> w571
        tunnel: w569 -> [w605 _]
        frame True {
          n208 = case shown="False" w605 {
            tunnel: w614 -> [w623 w755]
            tunnel: w613 -> [w622 w757]
            tunnel: w612 -> [w621 w758]
            tunnel: [w620 w752] -> w611
            tunnel: [w619 w751] -> w610
            tunnel: w609 -> [w618 w756]
            tunnel: [w617 w750] -> w608
            tunnel: w607 -> [w616 w754]
            tunnel: [w615 w753] -> w606
            frame False {
              n209 = case shown="10..33, 35..3F" w622 {
                selector: w622 -> [w634 w685 _]
                tunnel: w623 -> [w628 w687 w748]
                tunnel: w621 -> [w635 w686 _]
                tunnel: [w628 w683 w748] -> w620
                tunnel: [FALSE w679 FALSE] -> w619
                tunnel: w618 -> [w630 w681 _]
                tunnel: [w626 TRUE TRUE] -> w617
                tunnel: w616 -> [w627 w676 w746]
                tunnel: [w627 w675 w746] -> w615
                frame 16..51, 53..63 {
                  # "byte value from control parameters"
                  # "byte value from message"
                  # "check settings (don't change values)"
                  n210 = for {
                    tunnel: w635 -> [w672] mode=indexing
                    tunnel: w634 -> [w671]
                    shift-right: [w668] -> w633
                    shift-left: u8[] [] -> [w669]
                    # "find identifier in message"
                    n211 = Unbundle By Name(w672) -> ("Bytes"=w667:u8[], "Identifier"=w666:u8)
                    n212 = Equal?(x=w666, y=w671) -> (x = y?=w670:bool)
                    n213 = case shown="True" w670 {
                      tunnel: w669 -> [w673 _]
                      tunnel: [w673 w674] -> w668
                      tunnel: w667 -> [_ w674]
                      frame False {
                      }
                      frame True {
                      }
                    }
                  }
                  n214 = case shown="4" w630 {
                    tunnel: w633 -> [_ w642 w649 w657 w665]
                    tunnel: [u32 0 w638 w644 w651 w658] -> w632
                    frame Default {
                    }
                    frame 1 {
                      w637 = u8 0 ("hi")
                      n215 = Index Array(array=w642) -> (element=w641:u8)  [unwired: 1 in]
                      n216 = Join Numbers(hi=w637, lo=w637) -> ((hi.lo)=w640:u16)
                      n217 = Join Numbers(hi=w637, lo=w641) -> ((hi.lo)=w639:u16)
                      n218 = Join Numbers(hi=w640, lo=w639) -> ((hi.lo)=w638:u32)
                    }
                    frame 2 {
                      w643 = u8 0 ("hi")
                      n219 = Index Array(array=w649) -> (element #1=w648:u8, element #2=w647:u8)  [unwired: 2 in]
                      n220 = Join Numbers(hi=w643, lo=w643) -> ((hi.lo)=w646:u16)
                      n221 = Join Numbers(hi=w648, lo=w647) -> ((hi.lo)=w645:u16)
                      n222 = Join Numbers(hi=w646, lo=w645) -> ((hi.lo)=w644:u32)
                    }
                    frame 3 {
                      n223 = Index Array(array=w657) -> (element #1=w656:u8, element #2=w655:u8, element #3=w654:u8)  [unwired: 3 in]
                      n224 = Join Numbers(hi=u8 0, lo=w656) -> ((hi.lo)=w653:u16)
                      n225 = Join Numbers(hi=w655, lo=w654) -> ((hi.lo)=w652:u16)
                      n226 = Join Numbers(hi=w653, lo=w652) -> ((hi.lo)=w651:u32)
                    }
                    frame 4 {
                      n227 = Index Array(array=w665) -> (element #1=w664:u8, element #2=w663:u8, element #3=w662:u8, element #4=w661:u8)  [unwired: 4 in]
                      n228 = Join Numbers(hi=w664, lo=w663) -> ((hi.lo)=w660:u16)
                      n229 = Join Numbers(hi=w662, lo=w661) -> ((hi.lo)=w659:u16)
                      n230 = Join Numbers(hi=w660, lo=w659) -> ((hi.lo)=w658:u32)
                    }
                  }
                  n231 = Equal?(x=w632, y=w628) -> (x = y?=w626:bool)
                  n232 = Not(x=TRUE) -> (.not. x?=w625:bool)
                  n233 = Stop(stop? (T)=w625) -> ()
                }
                frame 52, 64, 65, 67..79 {
                  # "old aux byte value"
                  # "old byte value"
                  # "new byte value"
                  # "set front panel indicators"
                  n234 = for {
                    tunnel: w686 -> [w743] mode=indexing
                    tunnel: w685 -> [w742]
                    shift-right: [w739] -> w684
                    shift-left: u8[] [] -> [w740]
                    # "find identifier in message"
                    n235 = Unbundle By Name(w743) -> ("Bytes"=w738:u8[], "Identifier"=w737:u8)
                    n236 = Equal?(x=w737, y=w742) -> (x = y?=w741:bool)
                    n237 = case shown="True" w741 {
                      tunnel: w740 -> [w744 _]
                      tunnel: [w744 w745] -> w739
                      tunnel: w738 -> [_ w745]
                      frame False {
                      }
                      frame True {
                      }
                    }
                  }
                  n238 = case shown="1" w681 {
                    tunnel: w684 -> [_ w695 w703 w712 w721 w736]
                    tunnel: [w688 w691 w698 w706 w714 w723] -> w683
                    tunnel: [w688 w689 w696 w704 w713 w722] -> w675
                    tunnel: w676 -> [_ w689 w696 w704 w713 _]
                    frame Default {
                      w688 = u32 0
                    }
                    frame 1 {
                      w690 = u8 0 ("hi")
                      n239 = Index Array(array=w695) -> (element=w694:u8)  [unwired: 1 in]
                      n240 = Join Numbers(hi=w690, lo=w690) -> ((hi.lo)=w693:u16)
                      n241 = Join Numbers(hi=w690, lo=w694) -> ((hi.lo)=w692:u16)
                      n242 = Join Numbers(hi=w693, lo=w692) -> ((hi.lo)=w691:u32)
                    }
                    frame 2 {
                      w697 = u8 0 ("hi")
                      n243 = Index Array(array=w703) -> (element #1=w702:u8, element #2=w701:u8)  [unwired: 2 in]
                      n244 = Join Numbers(hi=w697, lo=w697) -> ((hi.lo)=w700:u16)
                      n245 = Join Numbers(hi=w702, lo=w701) -> ((hi.lo)=w699:u16)
                      n246 = Join Numbers(hi=w700, lo=w699) -> ((hi.lo)=w698:u32)
                    }
                    frame 3 {
                      n247 = Index Array(array=w712) -> (element #1=w711:u8, element #2=w710:u8, element #3=w709:u8)  [unwired: 3 in]
                      n248 = Join Numbers(hi=u8 0, lo=w711) -> ((hi.lo)=w708:u16)
                      n249 = Join Numbers(hi=w710, lo=w709) -> ((hi.lo)=w707:u16)
                      n250 = Join Numbers(hi=w708, lo=w707) -> ((hi.lo)=w706:u32)
                    }
                    frame 4 {
                      n251 = Index Array(array=w721) -> (element #1=w720:u8, element #2=w719:u8, element #3=w718:u8, element #4=w717:u8)  [unwired: 4 in]
                      n252 = Join Numbers(hi=w720, lo=w719) -> ((hi.lo)=w716:u16)
                      n253 = Join Numbers(hi=w718, lo=w717) -> ((hi.lo)=w715:u16)
                      n254 = Join Numbers(hi=w716, lo=w715) -> ((hi.lo)=w714:u32)
                    }
                    frame 8 {
                      n255 = Index Array(array=w736) -> (element #1=w735:u8, element #2=w734:u8, element #3=w733:u8, element #4=w732:u8, element #5=w727:u8, element #6=w726:u8, element #7=w725:u8, element #8=w724:u8)  [unwired: 8 in]
                      n256 = Join Numbers(hi=w735, lo=w734) -> ((hi.lo)=w731:u16)
                      n257 = Join Numbers(hi=w733, lo=w732) -> ((hi.lo)=w730:u16)
                      n258 = Join Numbers(hi=w727, lo=w726) -> ((hi.lo)=w729:u16)
                      n259 = Join Numbers(hi=w725, lo=w724) -> ((hi.lo)=w728:u16)
                      n260 = Join Numbers(hi=w731, lo=w730) -> ((hi.lo)=w722:u32)
                      n261 = Join Numbers(hi=w729, lo=w728) -> ((hi.lo)=w723:u32)
                    }
                  }
                  n262 = Not Equal?(x=w675, y=w676) -> (x != y?=w677:bool)
                  n263 = Not Equal?(x=w683, y=w687) -> (x != y?=w678:bool)
                  n264 = Or(x=w678, y=w677) -> (x .or. y?=w679:bool)
                }
                frame 66, Default {
                  (unwired) errorcluster {"status"=FALSE, "code"=0, "source"=""} ("error out")
                  (unwired) FALSE
                  # "GPS time stamp, default"
                }
              }
            }
            frame True {
              n265 = case shown="10..41, 43..4F" w757 {
                selector: w757 -> [w769 _]
                tunnel: w755 -> [w771 w832]
                tunnel: w758 -> [w770 _]
                tunnel: [w767 w832] -> w752
                tunnel: [w763 FALSE] -> w751
                tunnel: w756 -> [w765 _]
                tunnel: [TRUE TRUE] -> w750
                tunnel: w754 -> [w760 w830]
                tunnel: [w759 w830] -> w753
                frame 16..65, 67..79 {
                  # "old aux byte value"
                  # "old byte value"
                  # "new byte value"
                  # "set all values to device settings"
                  n266 = for {
                    tunnel: w770 -> [w827] mode=indexing
                    tunnel: w769 -> [w826]
                    shift-right: [w823] -> w768
                    shift-left: u8[] [] -> [w824]
                    # "find identifier in message"
                    n267 = Unbundle By Name(w827) -> ("Bytes"=w822:u8[], "Identifier"=w821:u8)
                    n268 = Equal?(x=w821, y=w826) -> (x = y?=w825:bool)
                    n269 = case shown="True" w825 {
                      tunnel: w824 -> [w828 _]
                      tunnel: [w828 w829] -> w823
                      tunnel: w822 -> [_ w829]
                      frame False {
                      }
                      frame True {
                      }
                    }
                  }
                  n270 = case shown="4" w765 {
                    tunnel: w768 -> [_ w779 w787 w796 w805 w820]
                    tunnel: [w772 w775 w782 w790 w798 w807] -> w767
                    tunnel: [w772 w773 w780 w788 w797 w806] -> w759
                    tunnel: w760 -> [_ w773 w780 w788 w797 _]
                    frame Default {
                      w772 = u32 0
                    }
                    frame 1 {
                      w774 = u8 0 ("hi")
                      n271 = Index Array(array=w779) -> (element=w778:u8)  [unwired: 1 in]
                      n272 = Join Numbers(hi=w774, lo=w774) -> ((hi.lo)=w777:u16)
                      n273 = Join Numbers(hi=w774, lo=w778) -> ((hi.lo)=w776:u16)
                      n274 = Join Numbers(hi=w777, lo=w776) -> ((hi.lo)=w775:u32)
                    }
                    frame 2 {
                      w781 = u8 0 ("hi")
                      n275 = Index Array(array=w787) -> (element #1=w786:u8, element #2=w785:u8)  [unwired: 2 in]
                      n276 = Join Numbers(hi=w781, lo=w781) -> ((hi.lo)=w784:u16)
                      n277 = Join Numbers(hi=w786, lo=w785) -> ((hi.lo)=w783:u16)
                      n278 = Join Numbers(hi=w784, lo=w783) -> ((hi.lo)=w782:u32)
                    }
                    frame 3 {
                      n279 = Index Array(array=w796) -> (element #1=w795:u8, element #2=w794:u8, element #3=w793:u8)  [unwired: 3 in]
                      n280 = Join Numbers(hi=u8 0, lo=w795) -> ((hi.lo)=w792:u16)
                      n281 = Join Numbers(hi=w794, lo=w793) -> ((hi.lo)=w791:u16)
                      n282 = Join Numbers(hi=w792, lo=w791) -> ((hi.lo)=w790:u32)
                    }
                    frame 4 {
                      n283 = Index Array(array=w805) -> (element #1=w804:u8, element #2=w803:u8, element #3=w802:u8, element #4=w801:u8)  [unwired: 4 in]
                      n284 = Join Numbers(hi=w804, lo=w803) -> ((hi.lo)=w800:u16)
                      n285 = Join Numbers(hi=w802, lo=w801) -> ((hi.lo)=w799:u16)
                      n286 = Join Numbers(hi=w800, lo=w799) -> ((hi.lo)=w798:u32)
                    }
                    frame 8 {
                      n287 = Index Array(array=w820) -> (element #1=w819:u8, element #2=w818:u8, element #3=w817:u8, element #4=w816:u8, element #5=w811:u8, element #6=w810:u8, element #7=w809:u8, element #8=w808:u8)  [unwired: 8 in]
                      n288 = Join Numbers(hi=w819, lo=w818) -> ((hi.lo)=w815:u16)
                      n289 = Join Numbers(hi=w817, lo=w816) -> ((hi.lo)=w814:u16)
                      n290 = Join Numbers(hi=w811, lo=w810) -> ((hi.lo)=w813:u16)
                      n291 = Join Numbers(hi=w809, lo=w808) -> ((hi.lo)=w812:u16)
                      n292 = Join Numbers(hi=w815, lo=w814) -> ((hi.lo)=w806:u32)
                      n293 = Join Numbers(hi=w813, lo=w812) -> ((hi.lo)=w807:u32)
                    }
                  }
                  n294 = Not Equal?(x=w759, y=w760) -> (x != y?=w761:bool)
                  n295 = Not Equal?(x=w767, y=w771) -> (x != y?=w762:bool)
                  n296 = Or(x=w762, y=w761) -> (x .or. y?=w763:bool)
                }
                frame 66, Default {
                  (unwired) errorcluster {"status"=FALSE, "code"=0, "source"=""} ("error out")
                  (unwired) FALSE
                  # "GPS time stamp, default"
                }
              }
            }
          }
        }
        frame False {
        }
      }
      n297 = Select(t=w575, s=w573, f=w573) -> (s? t:f=w576:bool)
    }
    frame "Slave" {
      n298 = case shown="\"Master\"" w855 {
        tunnel: [FALSE w863 w872] -> w856
        tunnel: w854 -> [_ w862 w871]
        tunnel: w853 -> [_ w861 w870]
        frame Default {
        }
        frame "Master" {
          n299 = String Subset(string=w862, length (rest)=3 ("length (rest)")) -> (substring=w866:string)  [unwired: 1 out]
          n300 = Not Equal?(x=Master."Slave", y=w861) -> (x != y?=w867:bool)
          n301 = Not Equal?(x=w866, y="SLV") -> (x != y?=w868:bool)
          n302 = And(x=w867, y=w868) -> (x .and. y?=w863:bool)
        }
        frame "Slave" {
          n303 = String Subset(string=w871, length (rest)=3 ("length (rest)")) -> (substring=w875:string)  [unwired: 1 out]
          n304 = Not Equal?(x=Master."Master", y=w870) -> (x != y?=w876:bool)
          n305 = Not Equal?(x=w875, y="MAS") -> (x != y?=w877:bool)
          n306 = And(x=w876, y=w877) -> (x .and. y?=w872:bool)
        }
      }
      n307 = case shown="True" w856 {
        tunnel: w858 -> [w887 w1107]
        tunnel: w847 -> [w886 _]
        tunnel: [w883 FALSE] -> w843
        tunnel: w857 -> [w885 _]
        tunnel: [w884 w1107] -> w852
        tunnel: w850 -> [w882 _]
        tunnel: [w881 TRUE] -> w846
        tunnel: w845 -> [w880 w1105]
        tunnel: [w879 w1105] -> w844
        tunnel: w842 -> [w878 _]
        frame True {
          n308 = case shown="False" w878 {
            tunnel: w887 -> [w896 w1026]
            tunnel: w886 -> [w895 w1028]
            tunnel: w885 -> [w894 w1029]
            tunnel: [w893 w1023] -> w884
            tunnel: [w892 w1022] -> w883
            tunnel: w882 -> [w891 w1027]
            tunnel: [w890 w1021] -> w881
            tunnel: w880 -> [w889 w1025]
            tunnel: [w888 w1024] -> w879
            frame False {
              n309 = case shown="10..33, 35..3F" w895 {
                selector: w895 -> [w905 w956 _]
                tunnel: w896 -> [w898 w958 w1019]
                tunnel: w894 -> [w906 w957 _]
                tunnel: [w898 w954 w1019] -> w893
                tunnel: [FALSE w950 FALSE] -> w892
                tunnel: w891 -> [w901 w952 _]
                tunnel: [w900 TRUE TRUE] -> w890
                tunnel: w889 -> [w897 w947 w1017]
                tunnel: [w897 w946 w1017] -> w888
                frame 16..51, 53..63 {
                  # "byte value from control parameters"
                  # "byte value from message"
                  # "check settings (don't change values)"
                  n310 = for {
                    tunnel: w906 -> [w943] mode=indexing
                    tunnel: w905 -> [w942]
                    shift-right: [w939] -> w904
                    shift-left: u8[] [] -> [w940]
                    # "find identifier in message"
                    n311 = Unbundle By Name(w943) -> ("Bytes"=w938:u8[], "Identifier"=w937:u8)
                    n312 = Equal?(x=w937, y=w942) -> (x = y?=w941:bool)
                    n313 = case shown="True" w941 {
                      tunnel: w940 -> [w944 _]
                      tunnel: [w944 w945] -> w939
                      tunnel: w938 -> [_ w945]
                      frame False {
                      }
                      frame True {
                      }
                    }
                  }
                  n314 = case shown="4" w901 {
                    tunnel: w904 -> [_ w913 w920 w928 w936]
                    tunnel: [u32 0 w909 w915 w922 w929] -> w903
                    frame Default {
                    }
                    frame 1 {
                      w908 = u8 0 ("hi")
                      n315 = Index Array(array=w913) -> (element=w912:u8)  [unwired: 1 in]
                      n316 = Join Numbers(hi=w908, lo=w908) -> ((hi.lo)=w911:u16)
                      n317 = Join Numbers(hi=w908, lo=w912) -> ((hi.lo)=w910:u16)
                      n318 = Join Numbers(hi=w911, lo=w910) -> ((hi.lo)=w909:u32)
                    }
                    frame 2 {
                      w914 = u8 0 ("hi")
                      n319 = Index Array(array=w920) -> (element #1=w919:u8, element #2=w918:u8)  [unwired: 2 in]
                      n320 = Join Numbers(hi=w914, lo=w914) -> ((hi.lo)=w917:u16)
                      n321 = Join Numbers(hi=w919, lo=w918) -> ((hi.lo)=w916:u16)
                      n322 = Join Numbers(hi=w917, lo=w916) -> ((hi.lo)=w915:u32)
                    }
                    frame 3 {
                      n323 = Index Array(array=w928) -> (element #1=w927:u8, element #2=w926:u8, element #3=w925:u8)  [unwired: 3 in]
                      n324 = Join Numbers(hi=u8 0, lo=w927) -> ((hi.lo)=w924:u16)
                      n325 = Join Numbers(hi=w926, lo=w925) -> ((hi.lo)=w923:u16)
                      n326 = Join Numbers(hi=w924, lo=w923) -> ((hi.lo)=w922:u32)
                    }
                    frame 4 {
                      n327 = Index Array(array=w936) -> (element #1=w935:u8, element #2=w934:u8, element #3=w933:u8, element #4=w932:u8)  [unwired: 4 in]
                      n328 = Join Numbers(hi=w935, lo=w934) -> ((hi.lo)=w931:u16)
                      n329 = Join Numbers(hi=w933, lo=w932) -> ((hi.lo)=w930:u16)
                      n330 = Join Numbers(hi=w931, lo=w930) -> ((hi.lo)=w929:u32)
                    }
                  }
                  n331 = Equal?(x=w903, y=w898) -> (x = y?=w900:bool)
                }
                frame 52, 64, 65, 67..79 {
                  # "old aux byte value"
                  # "old byte value"
                  # "new byte value"
                  # "set front panel indicators"
                  n332 = for {
                    tunnel: w957 -> [w1014] mode=indexing
                    tunnel: w956 -> [w1013]
                    shift-right: [w1010] -> w955
                    shift-left: u8[] [] -> [w1011]
                    # "find identifier in message"
                    n333 = Unbundle By Name(w1014) -> ("Bytes"=w1009:u8[], "Identifier"=w1008:u8)
                    n334 = Equal?(x=w1008, y=w1013) -> (x = y?=w1012:bool)
                    n335 = case shown="True" w1012 {
                      tunnel: w1011 -> [w1015 _]
                      tunnel: [w1015 w1016] -> w1010
                      tunnel: w1009 -> [_ w1016]
                      frame False {
                      }
                      frame True {
                      }
                    }
                  }
                  n336 = case shown="1" w952 {
                    tunnel: w955 -> [_ w966 w974 w983 w992 w1007]
                    tunnel: [w959 w962 w969 w977 w985 w994] -> w954
                    tunnel: [w959 w960 w967 w975 w984 w993] -> w946
                    tunnel: w947 -> [_ w960 w967 w975 w984 _]
                    frame Default {
                      w959 = u32 0
                    }
                    frame 1 {
                      w961 = u8 0 ("hi")
                      n337 = Index Array(array=w966) -> (element=w965:u8)  [unwired: 1 in]
                      n338 = Join Numbers(hi=w961, lo=w961) -> ((hi.lo)=w964:u16)
                      n339 = Join Numbers(hi=w961, lo=w965) -> ((hi.lo)=w963:u16)
                      n340 = Join Numbers(hi=w964, lo=w963) -> ((hi.lo)=w962:u32)
                    }
                    frame 2 {
                      w968 = u8 0 ("hi")
                      n341 = Index Array(array=w974) -> (element #1=w973:u8, element #2=w972:u8)  [unwired: 2 in]
                      n342 = Join Numbers(hi=w968, lo=w968) -> ((hi.lo)=w971:u16)
                      n343 = Join Numbers(hi=w973, lo=w972) -> ((hi.lo)=w970:u16)
                      n344 = Join Numbers(hi=w971, lo=w970) -> ((hi.lo)=w969:u32)
                    }
                    frame 3 {
                      n345 = Index Array(array=w983) -> (element #1=w982:u8, element #2=w981:u8, element #3=w980:u8)  [unwired: 3 in]
                      n346 = Join Numbers(hi=u8 0, lo=w982) -> ((hi.lo)=w979:u16)
                      n347 = Join Numbers(hi=w981, lo=w980) -> ((hi.lo)=w978:u16)
                      n348 = Join Numbers(hi=w979, lo=w978) -> ((hi.lo)=w977:u32)
                    }
                    frame 4 {
                      n349 = Index Array(array=w992) -> (element #1=w991:u8, element #2=w990:u8, element #3=w989:u8, element #4=w988:u8)  [unwired: 4 in]
                      n350 = Join Numbers(hi=w991, lo=w990) -> ((hi.lo)=w987:u16)
                      n351 = Join Numbers(hi=w989, lo=w988) -> ((hi.lo)=w986:u16)
                      n352 = Join Numbers(hi=w987, lo=w986) -> ((hi.lo)=w985:u32)
                    }
                    frame 8 {
                      n353 = Index Array(array=w1007) -> (element #1=w1006:u8, element #2=w1005:u8, element #3=w1004:u8, element #4=w1003:u8, element #5=w998:u8, element #6=w997:u8, element #7=w996:u8, element #8=w995:u8)  [unwired: 8 in]
                      n354 = Join Numbers(hi=w1006, lo=w1005) -> ((hi.lo)=w1002:u16)
                      n355 = Join Numbers(hi=w1004, lo=w1003) -> ((hi.lo)=w1001:u16)
                      n356 = Join Numbers(hi=w998, lo=w997) -> ((hi.lo)=w1000:u16)
                      n357 = Join Numbers(hi=w996, lo=w995) -> ((hi.lo)=w999:u16)
                      n358 = Join Numbers(hi=w1002, lo=w1001) -> ((hi.lo)=w993:u32)
                      n359 = Join Numbers(hi=w1000, lo=w999) -> ((hi.lo)=w994:u32)
                    }
                  }
                  n360 = Not Equal?(x=w946, y=w947) -> (x != y?=w948:bool)
                  n361 = Not Equal?(x=w954, y=w958) -> (x != y?=w949:bool)
                  n362 = Or(x=w949, y=w948) -> (x .or. y?=w950:bool)
                }
                frame 66, Default {
                  (unwired) errorcluster {"status"=FALSE, "code"=0, "source"=""} ("error out")
                  (unwired) FALSE
                  # "GPS time stamp, default"
                }
              }
            }
            frame True {
              n363 = case shown="10..29, 35" w1028 {
                selector: w1028 -> [w1040 _]
                tunnel: w1026 -> [w1042 w1103]
                tunnel: w1029 -> [w1041 _]
                tunnel: [w1038 w1103] -> w1023
                tunnel: [w1034 FALSE] -> w1022
                tunnel: w1027 -> [w1036 _]
                tunnel: [TRUE TRUE] -> w1021
                tunnel: w1025 -> [w1031 w1101]
                tunnel: [w1030 w1101] -> w1024
                frame 16..41, 53 {
                  # "old aux byte value"
                  # "old byte value"
                  # "new byte value"
                  # "set all values to device settings"
                  n364 = for {
                    tunnel: w1041 -> [w1098] mode=indexing
                    tunnel: w1040 -> [w1097]
                    shift-right: [w1094] -> w1039
                    shift-left: u8[] [] -> [w1095]
                    # "find identifier in message"
                    n365 = Unbundle By Name(w1098) -> ("Bytes"=w1093:u8[], "Identifier"=w1092:u8)
                    n366 = Equal?(x=w1092, y=w1097) -> (x = y?=w1096:bool)
                    n367 = case shown="True" w1096 {
                      tunnel: w1095 -> [w1099 _]
                      tunnel: [w1099 w1100] -> w1094
                      tunnel: w1093 -> [_ w1100]
                      frame False {
                      }
                      frame True {
                      }
                    }
                  }
                  n368 = case shown="4" w1036 {
                    tunnel: w1039 -> [_ w1050 w1058 w1067 w1076 w1091]
                    tunnel: [w1043 w1046 w1053 w1061 w1069 w1078] -> w1038
                    tunnel: [w1043 w1044 w1051 w1059 w1068 w1077] -> w1030
                    tunnel: w1031 -> [_ w1044 w1051 w1059 w1068 _]
                    frame Default {
                      w1043 = u32 0
                    }
                    frame 1 {
                      w1045 = u8 0 ("hi")
                      n369 = Index Array(array=w1050) -> (element=w1049:u8)  [unwired: 1 in]
                      n370 = Join Numbers(hi=w1045, lo=w1045) -> ((hi.lo)=w1048:u16)
                      n371 = Join Numbers(hi=w1045, lo=w1049) -> ((hi.lo)=w1047:u16)
                      n372 = Join Numbers(hi=w1048, lo=w1047) -> ((hi.lo)=w1046:u32)
                    }
                    frame 2 {
                      w1052 = u8 0 ("hi")
                      n373 = Index Array(array=w1058) -> (element #1=w1057:u8, element #2=w1056:u8)  [unwired: 2 in]
                      n374 = Join Numbers(hi=w1052, lo=w1052) -> ((hi.lo)=w1055:u16)
                      n375 = Join Numbers(hi=w1057, lo=w1056) -> ((hi.lo)=w1054:u16)
                      n376 = Join Numbers(hi=w1055, lo=w1054) -> ((hi.lo)=w1053:u32)
                    }
                    frame 3 {
                      n377 = Index Array(array=w1067) -> (element #1=w1066:u8, element #2=w1065:u8, element #3=w1064:u8)  [unwired: 3 in]
                      n378 = Join Numbers(hi=u8 0, lo=w1066) -> ((hi.lo)=w1063:u16)
                      n379 = Join Numbers(hi=w1065, lo=w1064) -> ((hi.lo)=w1062:u16)
                      n380 = Join Numbers(hi=w1063, lo=w1062) -> ((hi.lo)=w1061:u32)
                    }
                    frame 4 {
                      n381 = Index Array(array=w1076) -> (element #1=w1075:u8, element #2=w1074:u8, element #3=w1073:u8, element #4=w1072:u8)  [unwired: 4 in]
                      n382 = Join Numbers(hi=w1075, lo=w1074) -> ((hi.lo)=w1071:u16)
                      n383 = Join Numbers(hi=w1073, lo=w1072) -> ((hi.lo)=w1070:u16)
                      n384 = Join Numbers(hi=w1071, lo=w1070) -> ((hi.lo)=w1069:u32)
                    }
                    frame 8 {
                      n385 = Index Array(array=w1091) -> (element #1=w1090:u8, element #2=w1089:u8, element #3=w1088:u8, element #4=w1087:u8, element #5=w1082:u8, element #6=w1081:u8, element #7=w1080:u8, element #8=w1079:u8)  [unwired: 8 in]
                      n386 = Join Numbers(hi=w1090, lo=w1089) -> ((hi.lo)=w1086:u16)
                      n387 = Join Numbers(hi=w1088, lo=w1087) -> ((hi.lo)=w1085:u16)
                      n388 = Join Numbers(hi=w1082, lo=w1081) -> ((hi.lo)=w1084:u16)
                      n389 = Join Numbers(hi=w1080, lo=w1079) -> ((hi.lo)=w1083:u16)
                      n390 = Join Numbers(hi=w1086, lo=w1085) -> ((hi.lo)=w1077:u32)
                      n391 = Join Numbers(hi=w1084, lo=w1083) -> ((hi.lo)=w1078:u32)
                    }
                  }
                  n392 = Not Equal?(x=w1030, y=w1031) -> (x != y?=w1032:bool)
                  n393 = Not Equal?(x=w1038, y=w1042) -> (x != y?=w1033:bool)
                  n394 = Or(x=w1033, y=w1032) -> (x .or. y?=w1034:bool)
                }
                frame 66, Default {
                  (unwired) errorcluster {"status"=FALSE, "code"=0, "source"=""} ("error out")
                  (unwired) FALSE
                  # "GPS time stamp, default"
                }
              }
            }
          }
        }
        frame False {
        }
      }
      n395 = Select(t=w848, s=w846, f=w846) -> (s? t:f=w849:bool)
    }
  }
  "Status/Errors out" <- w1
  "Value Changed?" <- w4
  "Settings ok? out" <- w3
  "Run twice?" <- w2
  n396 = case shown="True" w28 {
    tunnel: "Control Parameter in" -> [w1109 w1116]
    tunnel: w30 -> [w1115 _]
    tunnel: [w1114 w1116] -> w10
    tunnel: w29 -> [w1113 _]
    tunnel: w27 -> [w1112 _]
    tunnel: w25 -> [w1111 _]
    tunnel: w26 -> [w1110 _]
    frame True {
      # "change value"
      n397 = Bundle By Name(cluster=w1109, "Byte Value"=w1115, "Min Real Value"=w1112, "dReal/dByte"=w1111, "Description"=w1110, "Aux Byte Value"=w1113) -> (w1114:T15)
    }
    frame False {
      # "don't change value"
    }
  }
  "Control Parameter out" <- w10
